vi "Text control 2 v1.8.vi"() -> ()   [LabVIEW 2016]
panel:
  in  "byte count":u32=64
  in  "Serial Settings:Serial End Mode for Reads":u16(ring)=2 items=["None", "LastBit", "TermChar"]
  in  "Timeout (ms)":u32=10000
  in  "Enable Termination\nChar (T)":bool=TRUE
  in  "Termination char\n(0xA = '\\n' = LF)\n(0xD = '\\r' = CR)":u8=13 format="%.0x"
  in  "flow control":u16(ring) items=["None"=0, "XON/XOFF"=1, "RTS/CTS"=2, "DTR/DSR"=4]
  in  "stop bits":u16(ring)=10 items=["1.0"=10, "1.5"=15, "2.0"=20]
  in  "parity":u16(ring) items=["None", "Odd", "Even", "Mark", "Space"]
  in  "data bits":u16=8 min=5 max=8 step=1
  in  "VISA resource name":refnum<visa-resource-name>="COM6"
  in  "baud rate":u32=9600
  out "Serial output":string
  out "error out":errorcluster
  in  "Units":bool
  out "Elapsed Time":dbl caption="Elapsed Time (s)"
  out "Ion vs time":cluster{"Y data in":dbl[], "X data in":dbl[]}[](graph)
  out "Ig":dbl format="%.2e"
  out "Id":dbl format="%.2e"
  out "Is":dbl format="%.2e"
  out "I vs Vg":cluster{"Y data in":dbl[], "X data in":dbl[]}[](graph)
  in  "Panel Controls 2":T1={"Emergency Stop"=refnum, "TransGraph Max"=1e-05, "Text/Graph (text=false)"=TRUE, "TransGraph Min"=1e-11} {"TransGraph Min" format="%.2e"; "TransGraph Max" format="%.2e"}
  out "Currently running:":string="#output s 0 0 0 -0.008 0.008 0.002"
  out "Lines left to run:":string
  in  "Standby":T2
  in  "Full Reset":bool
  in  "SMU4":cluster{"on/off":bool, "Voltage":dbl} {"Voltage" min=-100.0 max=100.0 format="%.2f"}
  in  "Source/Drain Range":u8(slide)=6 max=11 scale=0.0..11.0
  in  "Source/Drain\nRange mode":u16(ring) items=["Auto", "Limited", "Fixed"]
  in  "Gate Range":u8(slide)=6 max=11 scale=0.0..11.0
  in  "Gate Range\nmode":u16(ring) items=["Auto", "Limited", "Fixed"]
  in  "Gate":T3={"Gate Start"=0.0, "Gate Stop"=2.0, "Gate Step (linear only)"=1.0, "Gate Compliance"=0.0001, "Gate PComp"=0.0, "Range mode"=0, "Range"=6} {"Range" max=11 scale=0.0..11.0; "Range mode" items=["Auto", "Limited", "Fixed"]; "Gate PComp" format="%^.2e"; "Gate Compliance" format="%^.2e"; "Gate Step (linear only)" format="%^.4e"; "Gate Stop" format="%^.4e"; "Gate Start" format="%^.4e"}
  in  "Drain 2":T4={"Drain Start"=0.0, "Drain Stop"=2.0, "Drain Compliance"=0.0001, "Drain Step"=1.0, "Drain PComp"=0.0, "Range mode"=0, "Range"=6} {"Range" max=11 scale=0.0..11.0; "Range mode" items=["Auto", "Limited", "Fixed"]; "Drain PComp" format="%^.2e"; "Drain Step" format="%^.4e"; "Drain Compliance" format="%^.2e"; "Drain Stop" format="%^.4e"; "Drain Start" format="%^.4e"}
  in  "Timings 2":T5={"integration time"=0, "Short/Long integration time"=0.00064, "hold time (sec)"=0.0, "delay time (sec)"=0.0, "Step Time (0 disables)"=0.0, "sweep method"=0, "Pulse period"=0.005, "Base voltage"=0.0, "Pulse width"=0.0005} {"Pulse width" min=0.0005 max=0.1 step=0.0001 format="%.4f"; "Base voltage" format="%^.4e"; "Pulse period" min=0.005 max=1.0 step=0.0001 format="%.4f"; "sweep method" items=["Continuous", "Pulsed"]; "Step Time (0 disables)" format="%.2f"; "delay time (sec)" format="%.4f"; "hold time (sec)" format="%.4f"; "Short/Long integration time" format="%^.0e"; "integration time" scale=0.0..2.0}
  in  "Panel Controls":T6={"Emergency Stop"=refnum, "TransGraph Max"=1e-05, "Text/Graph (text=false)"=TRUE} {"TransGraph Max" format="%.2e"}
  in  "Interrupt run":bool
  in  "Drain: Compliance":dbl=0.001 format="%.8f"
  in  "Gate: Compliance":dbl=0.001 format="%.8f"
  out "Path":path=path "C:/users/rlp38/09Apr2009LTtesting/test2.txt"
  in  "hold time /s":dbl format="%.2f"
  in  "delay time /s":dbl format="%.2f"
  in  "integration time":u32(slide) max=2 step=1 scale=0.0..2.0
  in  "Integration time (short)":dbl=0.0019 min=8e-05 max=0.0019 step=8e-05 format="%^.0e"
  in  "Integration time (long)":dbl=0.32 min=0.04 max=2.0 step=0.02 format="%.2f"
  in  "Step delay /s":dbl format="%.2f"
  in  "Program":string="#pulsedstressV d 0.03 20 0 0.5 0.0827 5\n#\n#itime s\n#gaterangemode l\n#drainrangemode l\n#pulsed on 0.05 0 0.02\n#transfer d 1 -1 -0.1 -1 -1 0\n#wait-min 1\n#transfer d 1 -1 -0.1 -1 -1 0\n#output d 0 -1 -0.5 0 -1 -0.1\n#transfer d -10 40 1 5 40 35\n#transfer d -10 40 1 5 40 35\n#output d 0 40 20 0 40 1\n#\n#\n#sample 1 0.008 221 6 0.003\n#samplei 400e-6 200 6 0.002 0.1\n#vsu2pulse -10 4\n#\n#stressV 0.016 0.03 2e-4 0.1e-3 11\n#stressI 220e-7 0.08 15\n#transfer s -1 1 0.5 -0.005 0.005 0.005\n#output s 0 0 0 -0.008 0.008 0.002\n"
  # "Syntax:\nitime [s|m|l]\ngaterangemode [a|l|f]\ndrainrangemode [a|l|f]\npulsed [on|off] PulsePeriod(sec) PulseBaseVoltage PulseONWidth(sec)\nstandby [on l off]\nwait NumMilliseconds\nwait-min NumMinutes\n# texthere = comment\ntransfer [s|d] VgStart VgStop VgStep VdStart VdStop VdStep\noutput [s|d] VgStart VgStop VgStep VdStart VdStop VdStep\nsample Vg Vd NumSamples Time(s) SampleInterval(s)\nsamplei Idg NumSamples Time(s) SampleInterval(s) VDGcompliance\n# if in doubt use SampleInterval(s) = 0.004\nstressV VG VD IGcompliance IDcompliance Duration(sec)\nstressI IDG VDGcompliance Duration(sec)\nvsu2pulse Bias Duration(s)\npulsedstressV [s|d] VEstop VgON VgOFF Period(s) PulseONwidth(s) Vd\nsample-fpp Vg Vd NumSamples Time\nresample-fpp Vg Vd\ntransfer-fpp [s|d] VgStart VgStop VgStep VdStart VdStop VdStep\noutput-fpp [s|d] VgStart VgStop VgStep VdStart VdStop VdStep\nserial SerialPortCommand"
  # "Time"
  # "Sec"
  # "Min"
  # "100 samples is approx 13s with medium integration"
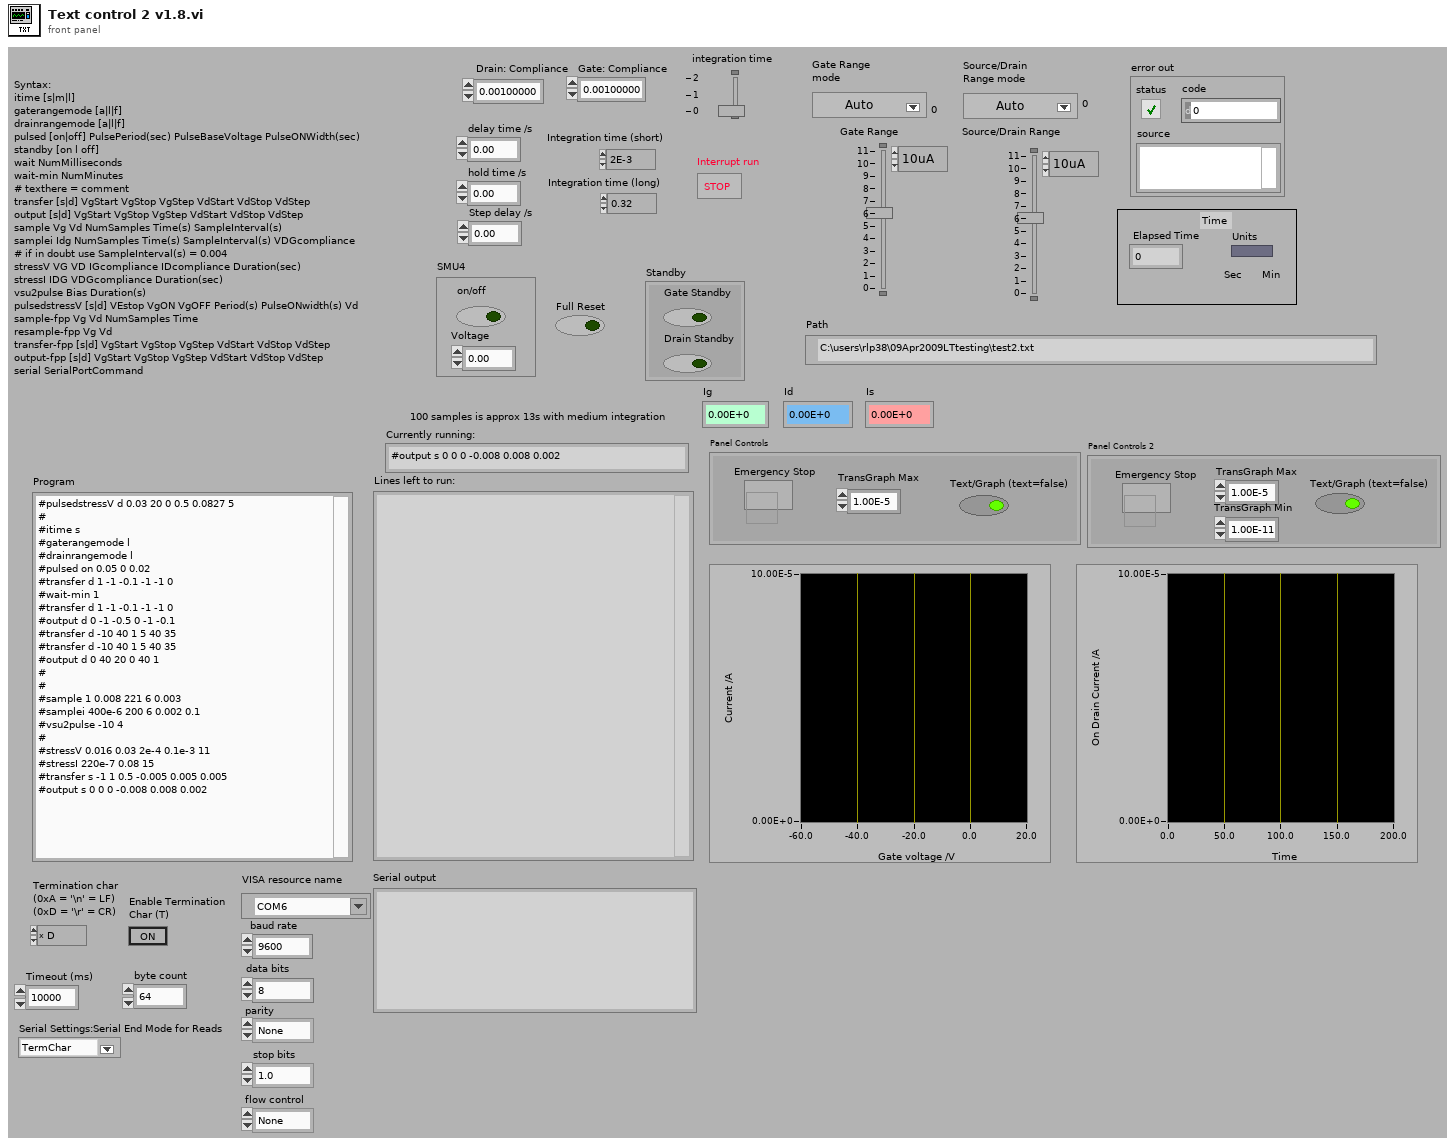
[diagram p1: front panel]
types:
  T1 = cluster{"Emergency Stop":refnum<vi>, "TransGraph Max":dbl, "Text/Graph (text=false)":bool, "TransGraph Min":dbl}
  T2 = cluster{"Gate Standby":bool, "Drain Standby":bool}
  T3 = cluster{"Gate Start":dbl, "Gate Stop":dbl, "Gate Step (linear only)":dbl, "Gate Compliance":dbl, "Gate PComp":dbl, "Range mode":u16, "Range":u8}
  T4 = cluster{"Drain Start":dbl, "Drain Stop":dbl, "Drain Compliance":dbl, "Drain Step":dbl, "Drain PComp":dbl, "Range mode":u16, "Range":u8}
  T5 = cluster{"integration time":u32, "Short/Long integration time":dbl, "hold time (sec)":dbl, "delay time (sec)":dbl, "Step Time (0 disables)":dbl, "sweep method":u16, "Pulse period":dbl, "Base voltage":dbl, "Pulse width":dbl}
  T6 = cluster{"Emergency Stop":refnum<vi>, "TransGraph Max":dbl, "Text/Graph (text=false)":bool}
  T7 = enum16{"open", "replace", "create", "open or create", "replace or create", "replace or create with confirmation"}
  T8 = cluster{"V2 Start":dbl, "V2 Step":dbl, "Number of points":i32}
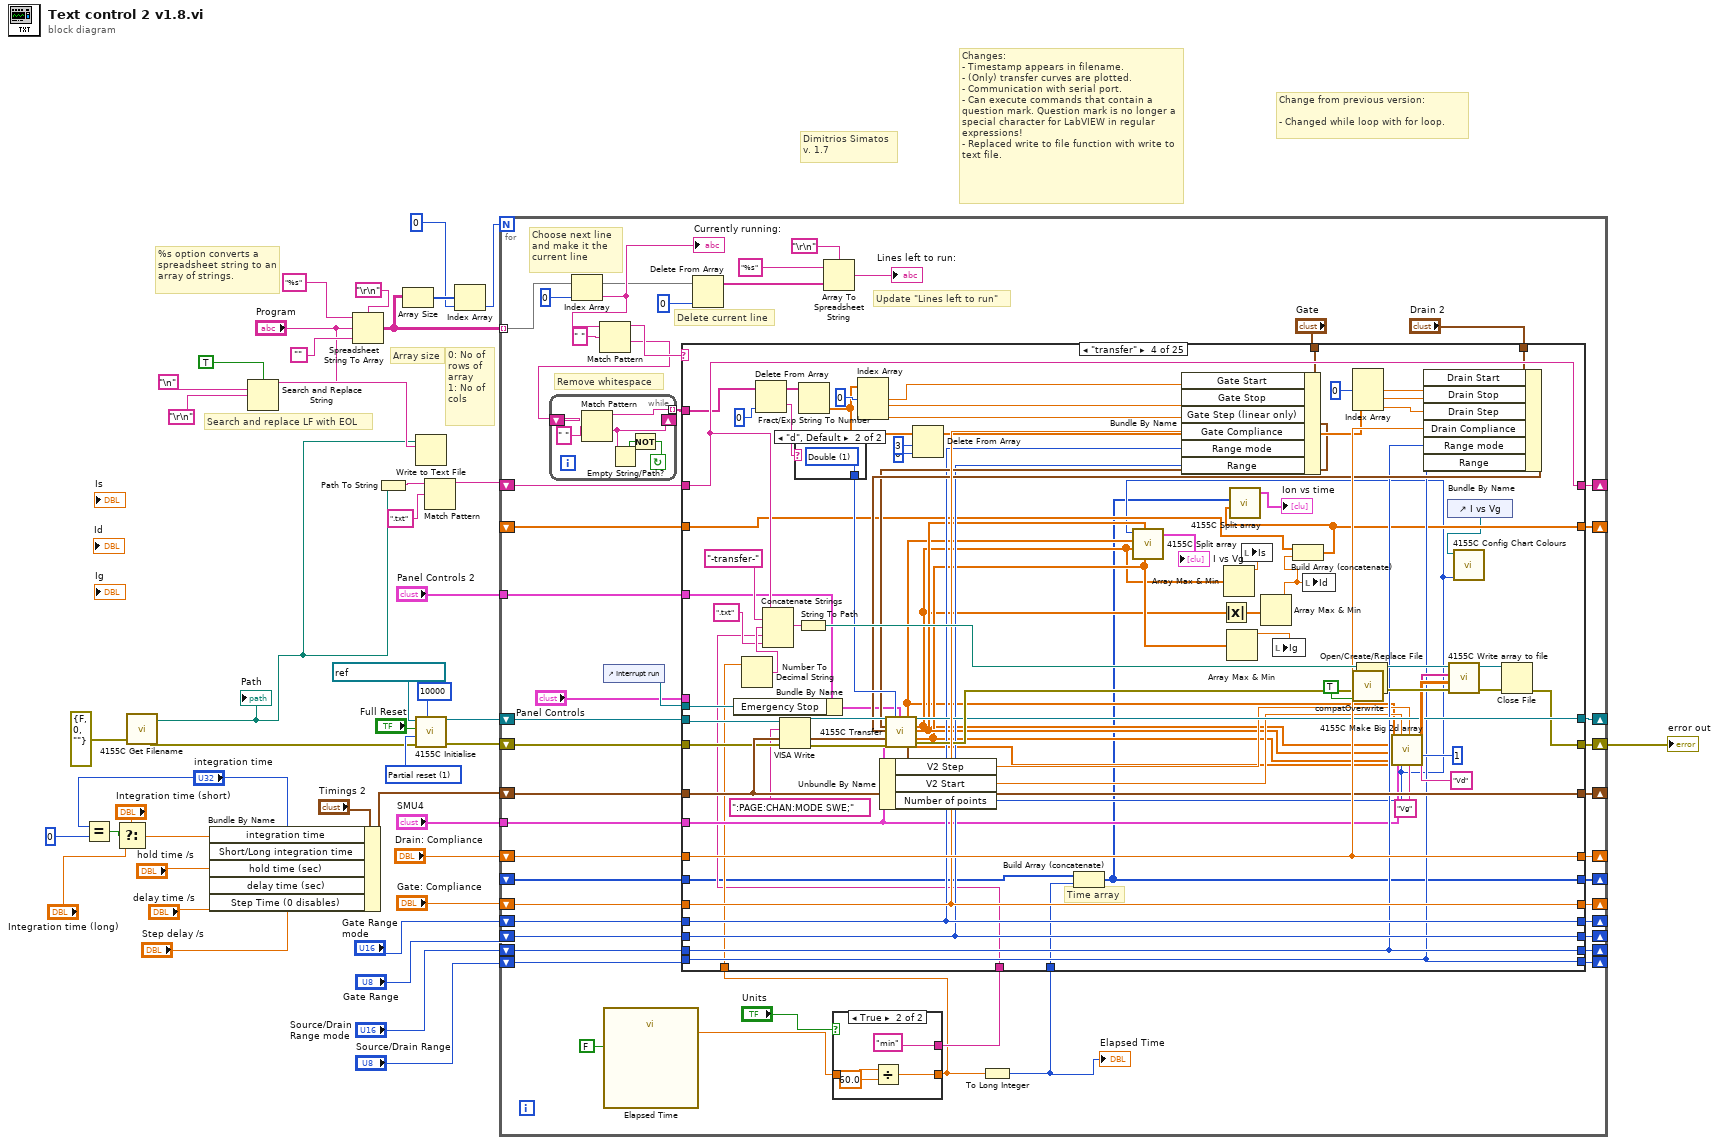
[diagram p0: block diagram]
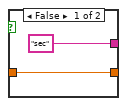
[diagram p2: hidden frame]
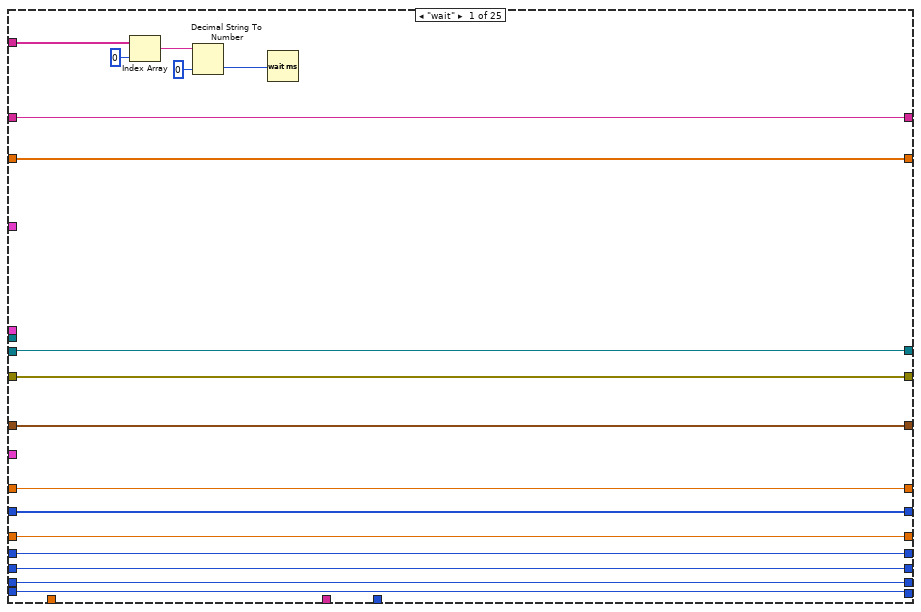
[diagram p3: hidden frame]
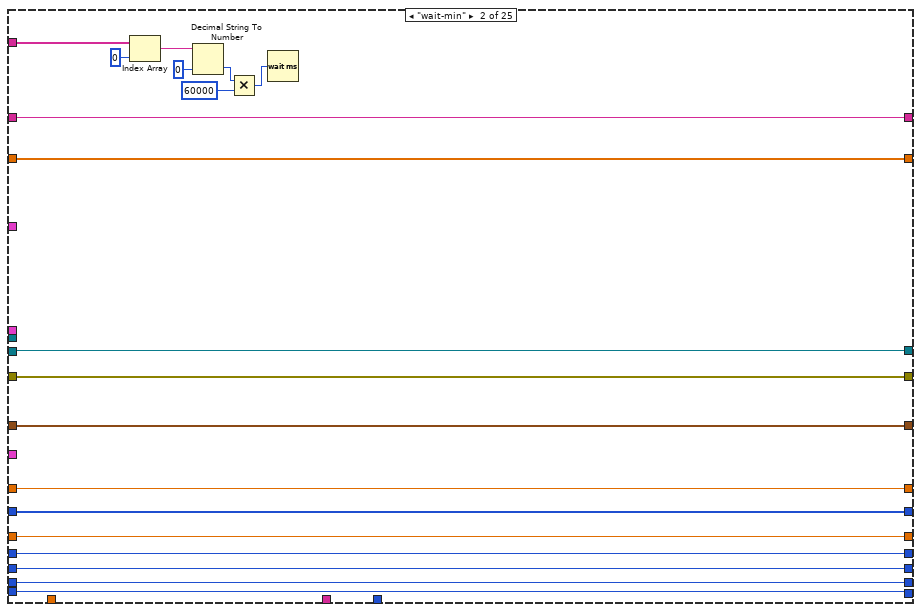
[diagram p4: hidden frame]
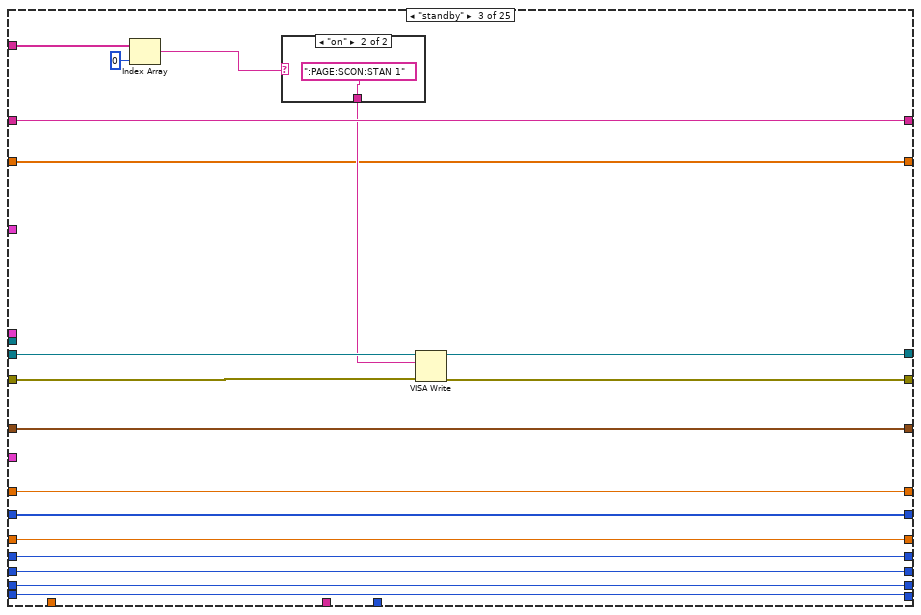
[diagram p5: hidden frame]
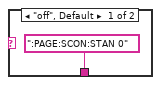
[diagram p6: hidden frame]
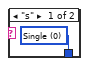
[diagram p7: hidden frame]
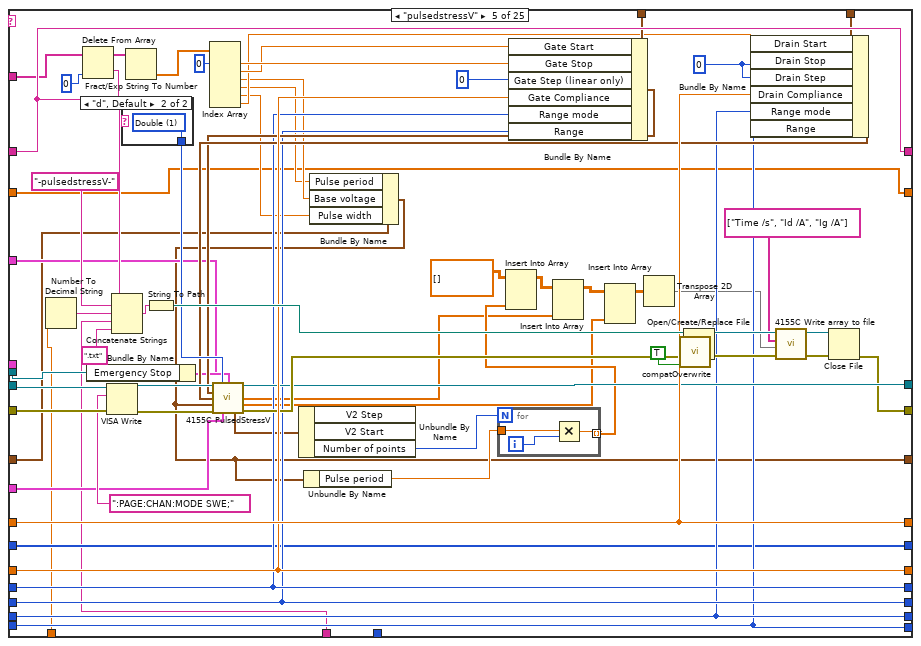
[diagram p8: hidden frame]
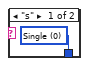
[diagram p9: hidden frame]
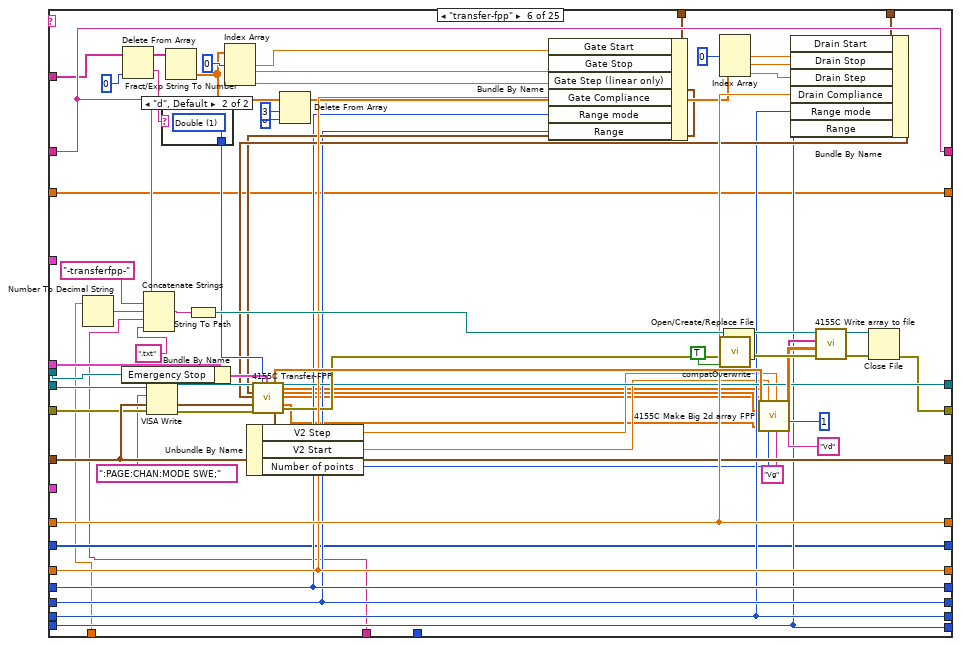
[diagram p10: hidden frame]
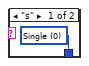
[diagram p11: hidden frame]
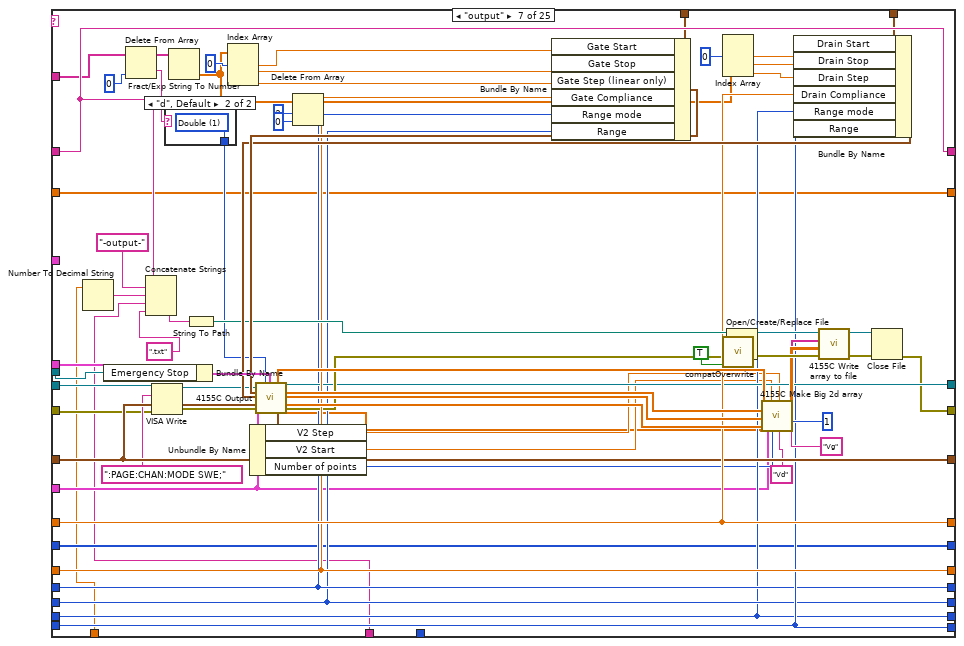
[diagram p12: hidden frame]
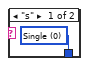
[diagram p13: hidden frame]
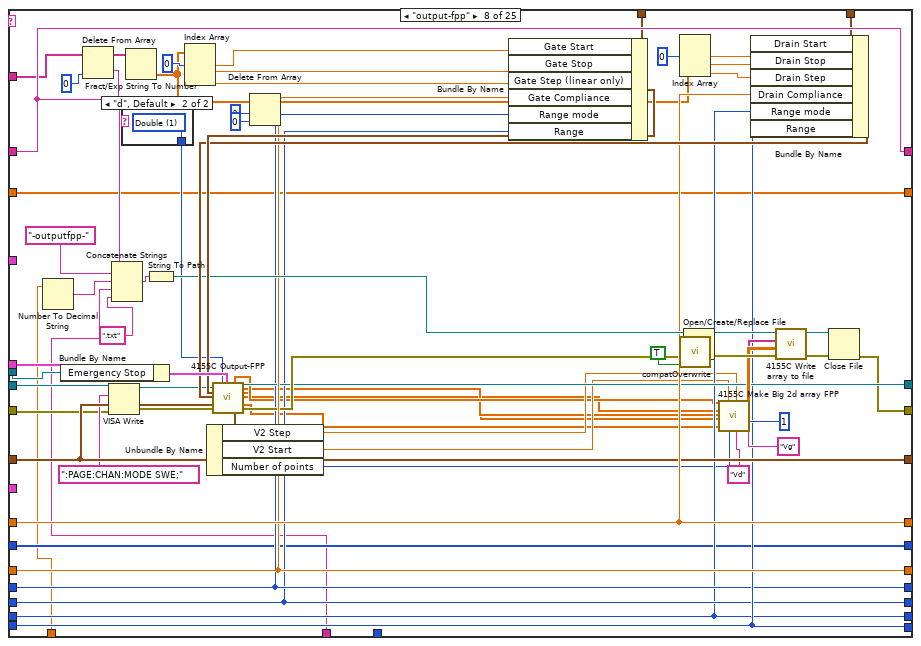
[diagram p14: hidden frame]
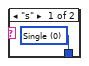
[diagram p15: hidden frame]
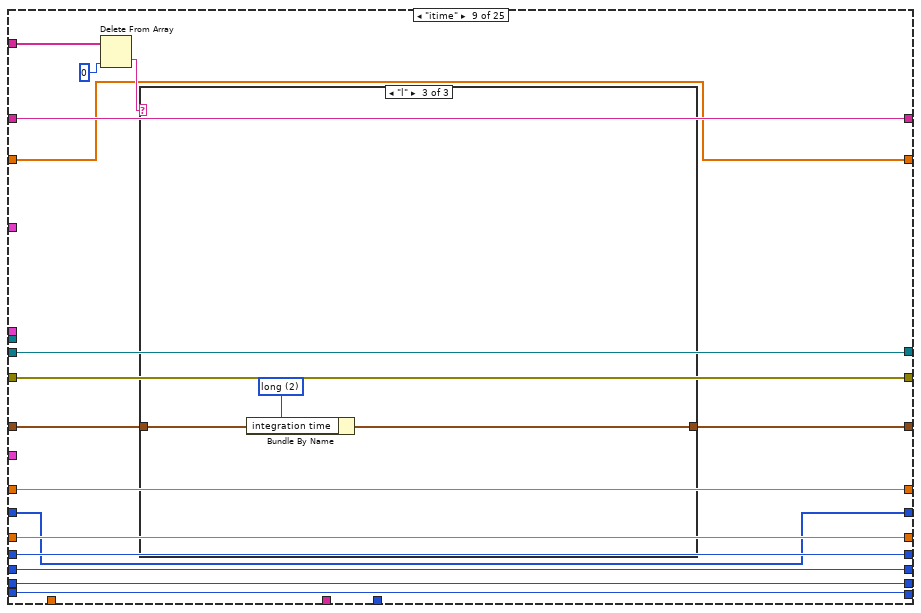
[diagram p16: hidden frame]
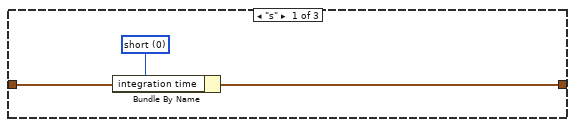
[diagram p17: hidden frame]
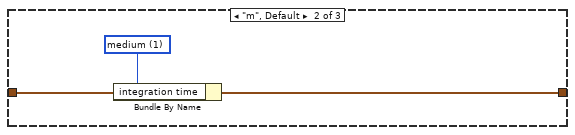
[diagram p18: hidden frame]
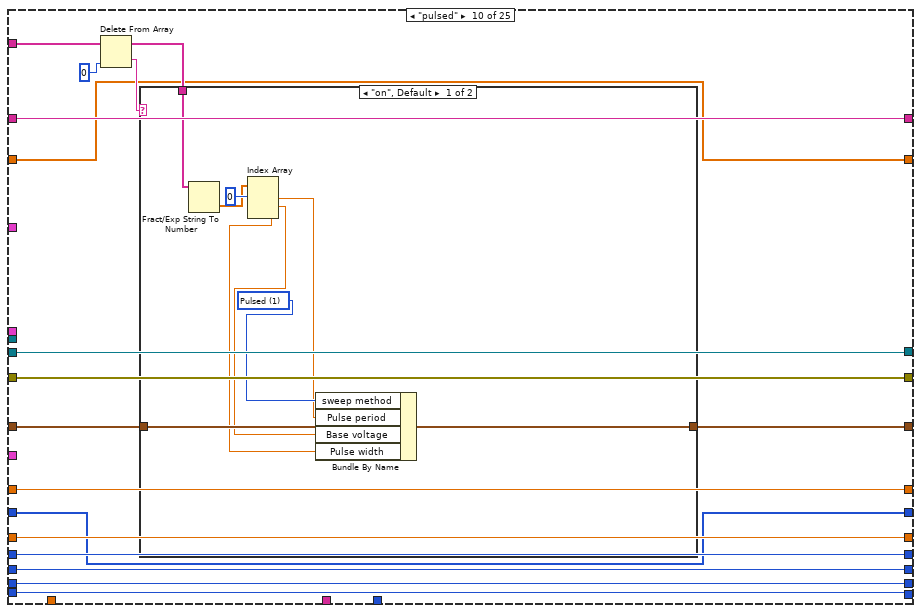
[diagram p19: hidden frame]
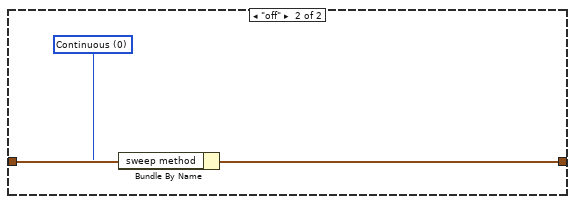
[diagram p20: hidden frame]
diagram:
  w35 = u16 1 items=["Reset All", "Partial reset"] ("Type of reset")
  # "Array size"
  # "%s option converts a spreadsheet string to an array of strings."
  # "0: No of rows of array\n1: No of cols"
  # "Change from previous version:\n\n- Changed while loop with for loop."
  # "Dimitrios Simatos\nv. 1.7"
  # "Changes:\n- Timestamp appears in filename.\n- (Only) transfer curves are plotted.\n- Communication with serial port.\n- Can execute commands that contain a question mark. Question mark is no longer a special character for LabVIEW in regular expressions!\n- Replaced write to file function with write to text file."
  # "Search and replace LF with EOL"
  n1 = Equal?(x="integration time", y=u32 0) -> (x = y?=w39:bool)
  n2 = Select(t="Integration time (short)", s=w39, f="Integration time (long)") -> (s? t:f=w43:dbl)
  n3 = call "4155C Get Filename.vi"("error in (no error)"=errorcluster {"status"=FALSE, "code"=0, "source"=""}) -> ("error out"=w30:errorcluster, "path"=w14:path)  [unwired: 2 in, 1 out]
  "Path" <- w14
  n4 = Bundle By Name(cluster="Timings 2", "integration time"="integration time", "Short/Long integration time"=w43, "hold time (sec)"="hold time /s", "delay time (sec)"="delay time /s", "Step Time (0 disables)"="Step delay /s") -> (w27:T5)
  n5 = Search and Replace String(replace all?=TRUE ("replace all? (F)"), input string="Program", search string="\n", replace string="\r\n") -> (result string=w17:string)  [unwired: 4 in, 3 out]
  n6 = Spreadsheet String To Array(delimiter (Tab)="\r\n", format string="%s", spreadsheet string="Program", array type (2D Dbl)="") -> (array=w2:string[][])
  n7 = Path To String(path=w14) -> (string=w13:string)
  n8 = Array Size(array=w2) -> (size(s)=w7:i32[])
  n9 = Write to Text File(file (use dialog)=w14, text=w17) -> ()  [unwired: 2 in, 3 out]
  n10 = call "4155C Initialise.vi"("VISA resource name in"=refnum<visa-resource-name> "GPIB0::14::INSTR", "Reset"="Full Reset", "Type of reset"=w35, "error in (no error)"=w30, "VISA Timeout Value"=u32 10000) -> ("VISA Resource Name out"=w29:refnum<visa-resource-name>, "error out"=w28:errorcluster)
  n11 = Match Pattern(string=w13, regular expression=".txt") -> (before substring=w12:string)  [unwired: 1 in, 3 out]
  n12 = Index Array(array=w7, index=0) -> (element=w5:i32)
  n13 = for {
    N: w5 -> [_]
    tunnel: "SMU4" -> [w64]
    shift-left: "Source/Drain Range" -> [w69]
    shift-right: [w65] -> _
    shift-left: "Source/Drain\nRange mode" -> [w70]
    shift-right: [w66] -> _
    shift-left: "Gate Range" -> [w71]
    shift-right: [w67] -> _
    shift-left: "Gate Range\nmode" -> [w72]
    shift-right: [w68] -> _
    shift-left: "Gate: Compliance" -> [w83]
    shift-right: [w78] -> _
    shift-left: "Drain: Compliance" -> [w84]
    shift-right: [w79] -> _
    shift-left: w27 -> [w85]
    shift-right: [w80] -> _
    shift-left: w28 -> [w86]
    shift-right: [w81] -> w9
    shift-left: w29 -> [w87]
    shift-right: [w82] -> _
    shift-left: w12 -> [w88]
    shift-right: [w77] -> _
    tunnel: "Panel Controls 2" -> [w63]
    shift-right: [w62] -> _
    shift-left: _ -> [w61]
    shift-right: [w56] -> _
    shift-left: _ -> [w55]
    tunnel: w2 -> [w51] mode=indexing
    # "Choose next line\nand make it the current line"
    # "Delete current line"
    # "Remove whitespace"
    # "Update \"Lines left to run\""
    n14 = Index Array(array=w51, index=0 ("line index")) -> (element=w52:string)
    "Currently running:" <- w52
    n15 = Match Pattern(string=w52, regular expression=" ") -> (before substring=w91:string, after substring=w90:string)  [unwired: 1 in, 2 out]
    n16 = while {
      tunnel: [w99] -> w89 mode=indexing
      shift-left: w90 -> [w101]
      shift-right: [w100] -> _
      stop <- w103 continue-if-true
      n17 = Match Pattern(string=w101, regular expression=" ") -> (before substring=w99:string, after substring=w100:string)  [unwired: 1 in, 2 out]
      n18 = Empty String/Path?(string/path=w100) -> (empty?=w104:bool)
      n19 = Not(x=w104) -> (.not. x?=w103:bool)
    }
    n20 = control-ref of="Interrupt run"() -> (w76:refnum<vi>)
    n21 = call "Elapsed Time"("Auto Reset"=FALSE) -> ("Elapsed Time (s)"=w57:dbl)  [unwired: 11 in, 7 out]
    n22 = Delete From Array(array=w51, index=0) -> (array with subset deleted=w50:string[])  [unwired: 1 in, 1 out]
    n23 = Array To Spreadsheet String(delimiter (Tab)="\r\n", array=w50, 3:"%s" ("format string")) -> (spreadsheet string=→"Lines left to run:":string)
    n24 = case shown="True" "Units" {
      tunnel: ["sec" "min"] -> w58
      tunnel: [w93 w97] -> w54
      tunnel: w57 -> [w93 w96]
      frame False {
      }
      frame True {
        n25 = Divide(x=w96, y=60.0) -> (x/y=w97:dbl)
      }
    }
    n26 = To Long Integer(number=w54) -> (32bit integer=w53:i32)
    "Elapsed Time" <- w53
    n27 = case shown="\"transfer\"" w91 {
      tunnel: w89 -> [w121 w140 w158 w222 w293 w362 w429 w504 w542 w568 w595 w620 w641 w655 _ _ w759 w820 _ w885 w929 w971 w1041 w1103 w1110]
      tunnel: w88 -> [w116 w136 w156 w230 w300 w370 w437 w512 w531 w557 w587 w613 w635 w648 w667 w709 w737 w802 w833 w872 w916 w959 w1035 w1099 w1112]
      tunnel: w87 -> [w115 w135 w147 w200 w284 w339 w405 w480 w532 w558 w588 w614 w636 w649 w672 w711 w765 w826 w837 w891 w935 w977 w1047 w1057 w1116]
      tunnel: w86 -> [w114 w134 w146 w199 w283 w338 w402 w477 w533 w559 w589 w615 w637 w650 w671 w682 w764 w825 w836 w890 w934 w976 w1046 w1056 w1115]
      tunnel: w85 -> [w113 w133 w155 w226 w259 w366 w433 w508 w541 w567 w586 w612 w634 w647 w670 w706 w728 w794 w842 w865 w909 w952 w1034 w1098 w1117]
      tunnel: w84 -> [w112 w132 w154 w228 w298 w368 w435 w510 w540 w566 w594 w619 w640 w654 w669 w691 w763 w824 w845 w889 w933 w975 w1045 w1107 w1118]
      tunnel: w83 -> [w111 w131 w153 w227 w297 w367 w434 w509 w539 w565 w593 w618 w639 w653 w668 w692 w738 w803 w844 w873 w917 w960 w1036 w1100 w1120]
      tunnel: [w115 w135 w145 w224 w295 w364 w431 w506 w532 w558 w588 w614 w636 w649 w672 w711 w729 w776 w835 w866 w910 w953 w987 w1059 w1116] -> w82
      tunnel: [w114 w134 w144 w223 w294 w363 w430 w505 w533 w559 w589 w615 w637 w650 w671 w681 w739 w777 w834 w874 w918 w961 w986 w1058 w1114] -> w81
      tunnel: [w113 w133 w155 w226 w255 w366 w433 w508 w534 w560 w586 w612 w634 w647 w670 w706 w728 w794 w842 w865 w909 w952 w1034 w1098 w1117] -> w80
      tunnel: [w112 w132 w154 w228 w298 w368 w435 w510 w540 w566 w594 w619 w640 w654 w669 w691 w763 w824 w845 w889 w933 w975 w1045 w1107 w1118] -> w79
      tunnel: [w111 w131 w153 w227 w297 w367 w434 w509 w539 w565 w593 w618 w639 w653 w668 w692 w738 w803 w844 w873 w917 w960 w1036 w1100 w1120] -> w78
      tunnel: [w116 w136 w156 w230 w300 w370 w437 w512 w531 w557 w587 w613 w635 w648 w667 w709 w737 w802 w833 w872 w916 w959 w1035 w1099 w1112] -> w77
      tunnel: w76 -> [_ _ _ w233 w304 w375 w445 w516 _ _ _ _ _ _ _ _ w734 w799 _ w871 w915 w958 w1007 w1075 _]
      tunnel: "Gate" -> [_ _ _ w209 w287 w349 w416 w491 _ _ _ _ _ _ _ _ _ _ _ _ _ _ _ _ _]
      tunnel: "Drain 2" -> [_ _ _ w208 w286 w348 w415 w490 _ _ _ _ _ _ _ _ _ _ _ _ _ _ _ _ _]
      tunnel: "Panel Controls" -> [_ _ _ _ _ w347 w414 w489 _ _ _ _ _ _ _ _ _ _ _ _ _ _ _ _ _]
      tunnel: w72 -> [w110 w130 w152 w193 w277 w332 w400 w475 w538 w564 _ w611 w633 w646 w666 w693 w724 w790 w838 w861 w905 w948 w1030 w1094 w1121]
      tunnel: w71 -> [w109 w129 w151 w192 w276 w331 w399 w474 w537 w563 w592 _ w624 w652 w665 w694 w725 w791 w839 w862 w906 w949 w1031 w1095 w1122]
      tunnel: w70 -> [w108 w128 w150 w191 w275 w330 w398 w473 w536 w562 w591 w617 w638 _ w664 w695 w726 w792 w840 w863 w907 w950 w1032 w1096 w1123]
      tunnel: w69 -> [w107 w127 w149 w190 w274 w329 w401 w476 w535 w561 w590 w616 _ w651 w663 w696 w727 w793 w841 w864 w908 w951 w1033 w1097 w1124]
      tunnel: [w110 w130 w152 w193 w277 w332 w400 w475 w538 w564 w585 w611 w633 w646 w666 w693 w724 w790 w838 w861 w905 w948 w1030 w1094 w1121] -> w68
      tunnel: [w109 w129 w151 w192 w276 w331 w399 w474 w537 w563 w592 w603 w624 w652 w665 w694 w725 w791 w839 w862 w906 w949 w1031 w1095 w1122] -> w67
      tunnel: [w108 w128 w150 w191 w275 w330 w398 w473 w536 w562 w591 w617 w638 w645 w664 w695 w726 w792 w840 w863 w907 w950 w1032 w1096 w1123] -> w66
      tunnel: [w107 w127 w149 w190 w274 w329 w401 w476 w535 w561 w590 w616 w625 w651 w663 w696 w727 w793 w841 w864 w908 w951 w1033 w1097 w1124] -> w65
      tunnel: w64 -> [_ _ _ w185 w271 _ w393 _ _ _ _ _ _ _ _ _ _ _ _ _ _ _ _ _ _]
      tunnel: w63 -> [_ _ _ w183 w270 _ _ _ _ _ _ _ _ _ _ _ _ _ _ _ _ _ _ _ _]
      tunnel: [w106 w123 w142 w172 w247 w319 w390 w462 w530 w555 w584 w602 w623 w644 w662 w677 w716 w774 w832 w850 w898 w942 w984 w1052 w1113] -> w62
      tunnel: w61 -> [w106 w123 w142 w171 w247 w319 w390 w462 w530 w555 w584 w602 w623 w644 w662 w677 w716 w774 w832 w850 w898 w942 w984 w1052 w1113]
      tunnel: w54 -> [_ _ _ w167 w244 w317 w387 w459 _ _ _ _ _ _ _ w675 w714 w771 _ w847 w895 w939 w981 w1048 _]
      tunnel: w58 -> [_ _ _ w164 w243 w315 w386 w458 _ _ _ _ _ _ _ w673 w712 w770 _ w846 w894 w938 w980 w1049 _]
      tunnel: w53 -> [_ _ _ w161 _ _ _ _ _ _ _ _ _ _ _ _ _ _ _ _ _ _ _ _ _]
      tunnel: [w105 w122 w141 w163 w246 w318 w389 w461 w529 w554 w583 w601 w622 w643 w661 w676 w715 w773 w831 w849 w897 w941 w983 w1051 w1119] -> w56
      tunnel: w55 -> [w105 w122 w141 w162 w246 w318 w389 w461 w529 w554 w583 w601 w622 w643 w661 w676 w715 w773 w831 w849 w897 w941 w983 w1051 w1119]
      frame "wait" {
        n28 = Index Array(array=w121, index=0 ("Index")) -> (element=w119:string)
        n29 = Decimal String To Number(string=w119, default (0L)=u32 0) -> (number=w118:u32)  [unwired: 1 in, 1 out]
        n30 = Wait (ms)(milliseconds to wait=w118) -> ()  [unwired: 1 out]
      }
      frame "wait-min" {
        n31 = Index Array(array=w140, index=0 ("Index")) -> (element=w138:string)
        n32 = Decimal String To Number(string=w138, default (0L)=u32 0) -> (number=w126:u32)  [unwired: 1 in, 1 out]
        n33 = Multiply(x=w126, y=u32 60000) -> (x*y=w125:u32)
        n34 = Wait (ms)(milliseconds to wait=w125) -> ()  [unwired: 1 out]
      }
      frame "standby" {
        n35 = Index Array(array=w158, index=0 ("Index")) -> (element=w148:string)
        n36 = case shown="\"on\"" w148 {
          tunnel: [":PAGE:SCON:STAN 0" ":PAGE:SCON:STAN 1"] -> w143
          frame "off", Default {
          }
          frame "on" {
          }
        }
        n37 = VISA Write(VISA resource name=w147, write buffer=w143, error in (no error)=w146) -> (VISA resource name out=w145:refnum<visa-resource-name>, error out=w144:errorcluster)  [unwired: 1 out]
      }
      frame "transfer" {
        # "Time array"
        n38 = Bundle By Name(cluster=w183, "Emergency Stop"=w233) -> (w184:T1)
        n39 = Number To Decimal String(number=w167) -> (decimal integer string=w166:string)  [unwired: 1 in]
        n40 = Delete From Array(array=w222, index=0 ("Index")) -> (deleted portion=w220:string, array with subset deleted=w219:string[])  [unwired: 1 in]
        n41 = Concatenate Strings(w230, "-transfer-" ("Prefix"), w166, w164, ".txt" ("Suffix")) -> (w232:string)
        n42 = VISA Write(VISA resource name=w200, write buffer=":PAGE:CHAN:MODE SWE;" ("write buffer (\"\")"), error in (no error)=w199) -> (VISA resource name out=w197:refnum<visa-resource-name>, error out=w198:errorcluster)  [unwired: 1 out]
        n43 = case shown="\"d\", Default" w220 {
          tunnel: [w241 w242] -> w218
          frame "s" {
            w241 = u16 0 items=["Single", "Double"] ("sweep mode")
          }
          frame "d", Default {
            w242 = u16 1 items=["Single", "Double"] ("sweep mode")
          }
        }
        n44 = String To Path(string=w232) -> (path=w229:path)
        n45 = Fract/Exp String To Number(string=w219) -> (number=w204:dbl[])  [unwired: 3 in, 1 out]
        n46 = Index Array(array=w204, index #1=0 ("Index")) -> (element #1=w217:dbl, element #2=w216:dbl, element #3=w215:dbl)  [unwired: 2 in]
        n47 = Delete From Array(array=w204, length=3 ("Length"), index=0 ("Index")) -> (array with subset deleted=w202:dbl[])  [unwired: 1 out]
        n48 = Build Array (concatenate)(w162, w161) -> (w163:i32[])
        n49 = Bundle By Name(cluster=w209, "Gate Start"=w217, "Gate Stop"=w216, "Gate Step (linear only)"=w215, "Gate Compliance"=w227, "Range mode"=w193, "Range"=w192) -> (w194:T3)
        n50 = Index Array(array=w202, index #1=0 ("Index")) -> (element #1=w212:dbl, element #2=w211:dbl, element #3=w210:dbl)  [unwired: 2 in]
        n51 = call <vilib>:"compatOverwrite.vi"("overwrite (F)"=TRUE) -> ("overwrite?"=w182:T7)
        n52 = Bundle By Name(cluster=w208, "Drain Start"=w212, "Drain Stop"=w211, "Drain Step"=w210, "Drain Compliance"=w228, "Range mode"=w191, "Range"=w190) -> (w195:T4)
        n53 = call "4155C Transfer.vi"("VISA resource name in"=w197, "Gate"=w194, "Drain"=w195, "Timings"=w226, "error in (no error)"=w198, "SMU4"=w185, "sweep mode"=w218, "Panel Controls"=w184) -> ("VG"=w173:dbl[], "Outparams"=w189:T8, "VISA Resource Name out"=w224:refnum<visa-resource-name>, "IS"=w175:dbl[], "ID"=w180:dbl[], "IG"=w176:dbl[], "error out"=w225:errorcluster, "SMU4"=w186:dbl[])  [unwired: 12 in]
        n54 = Unbundle By Name(w189) -> ("V2 Step"=w188:dbl, "V2 Start"=w187:dbl, "Number of points"=w169:i32)
        n55 = call "4155C Split array.vi"("Number of VAR2 steps"=w169, "Y2 data in"=w180, "X data in"=w173, "Y1 data in"=w175, "Y3 data in"=w176) -> ("Array of clusters"=→"I vs Vg":cluster{"Y data in":dbl[], "X data in":dbl[]}[])  [unwired: 2 in, 1 out]
        n56 = Absolute Value(x=w175) -> (abs(x)=w179:dbl[])
        n57 = Array Max & Min(array=w175) -> (max value=w177:dbl)  [unwired: 3 out]
        n58 = Array Max & Min(array=w176) -> (max value=w178:dbl)  [unwired: 3 out]
        n59 = local write "Is"(w177) -> ()
        n60 = Array Max & Min(array=w179) -> (max value=w170:dbl)  [unwired: 3 out]
        n61 = local write "Ig"(w178) -> ()
        n62 = Build Array (concatenate)(w171, w170) -> (w172:dbl[])
        n63 = call "4155C Split array.vi"("X data in"=w163, "Y1 data in"=w172) -> ("Array of clusters"=→"Ion vs time":cluster{"Y data in":dbl[], "X data in":dbl[]}[])  [unwired: 5 in, 1 out]
        n64 = local write "Id"(w170) -> ()
        n65 = Open/Create/Replace File(file path (use dialog)=w229, error in=w225, operation (0:open)=w182) -> (refnum out=w238:refnum<file>, error out=w239:errorcluster)  [unwired: 3 in, 1 out]
        n66 = call "4155C Make Big 2d array.vi"("1D Var1"=w173, "1d IS"=w175, "1d ID"=w180, "1d IG"=w176, "1d SMU4"=w186, "SMU4"=w185, "VAR2 START"=w187, "Number of VAR2 steps"=w169, "VAR2 STEP"=w188, "VAR1 Name"="Vg", "Decimal places in header"=i8 1, "VAR2 Name"="Vd") -> ("Header array"=w234:string[], "Data array"=w235:dbl[][])  [unwired: 14 in]
        n67 = control-ref of="I vs Vg"() -> (w168:refnum<vi>)
        n68 = call "4155C Write array to file.vi"("Byte Stream File Refnum"=w238, "Header"=w234, "Data Array"=w235, "error in (no error)"=w239) -> ("dup refnum"=w236:refnum<file>, "error out"=w237:errorcluster)  [unwired: 1 in]
        n69 = call "4155C Config Chart Colours.vi"("Numeric"=w169, "XY Graph 2"=w168) -> ()  [unwired: 6 in]
        n70 = Close File(refnum=w236, error in=w237) -> (error out=w223:errorcluster)  [unwired: 1 out]
      }
      frame "pulsedstressV" {
        w253 = 0
        n71 = Number To Decimal String(number=w244) -> (decimal integer string=w301:string)  [unwired: 1 in]
        n72 = Delete From Array(array=w293, index=0 ("Index")) -> (deleted portion=w291:string, array with subset deleted=w290:string[])  [unwired: 1 in]
        n73 = Bundle By Name(cluster=w270, "Emergency Stop"=w304) -> (w272:T1)
        n74 = VISA Write(VISA resource name=w284, write buffer=":PAGE:CHAN:MODE SWE;" ("write buffer (\"\")"), error in (no error)=w283) -> (VISA resource name out=w281:refnum<visa-resource-name>, error out=w282:errorcluster)  [unwired: 1 out]
        n75 = Concatenate Strings(w300, "-pulsedstressV-" ("Substring"), w301, w243, ".txt" ("Substring")) -> (w303:string)
        n76 = case shown="\"d\", Default" w291 {
          tunnel: [w313 w314] -> w289
          frame "s" {
            w313 = u16 0 items=["Single", "Double"] ("sweep mode")
          }
          frame "d", Default {
            w314 = u16 1 items=["Single", "Double"] ("sweep mode")
          }
        }
        n77 = Fract/Exp String To Number(string=w290) -> (number=w285:dbl[])  [unwired: 3 in, 1 out]
        n78 = String To Path(string=w303) -> (path=w299:path)
        n79 = Index Array(array=w285, index #1=0 ("Index")) -> (element #1=w262:dbl, element #2=w261:dbl, element #3=w258:dbl, element #4=w257:dbl, element #5=w256:dbl, element #6=w260:dbl)  [unwired: 5 in]
        n80 = Bundle By Name(cluster=w259, "Pulse period"=w257, "Base voltage"=w258, "Pulse width"=w256) -> (w255:T5)
        n81 = Unbundle By Name(w255) -> ("Pulse period"=w263:dbl)
        n82 = Bundle By Name(cluster=w287, "Gate Start"=w261, "Gate Stop"=w262, "Gate Step (linear only)"=0, "Gate Compliance"=w297, "Range mode"=w277, "Range"=w276) -> (w278:T3)
        n83 = call <vilib>:"compatOverwrite.vi"("overwrite (F)"=TRUE) -> ("overwrite?"=w248:T7)
        n84 = Bundle By Name(cluster=w286, "Drain Start"=w260, "Drain Stop"=w253, "Drain Step"=w253, "Drain Compliance"=w298, "Range mode"=w275, "Range"=w274) -> (w279:T4)
        n85 = call "4155C PulsedStressV.vi"("VISA resource name in"=w281, "sweep mode"=w289, "Panel Controls"=w272, "Gate"=w278, "Drain"=w279, "Timings"=w255, "error in (no error)"=w282, "SMU4"=w271) -> ("VISA Resource Name out"=w295:refnum<visa-resource-name>, "ID"=w251:dbl[], "IG"=w249:dbl[], "Outparams"=w273:T8, "error out"=w296:errorcluster)  [unwired: 3 in]
        n86 = Unbundle By Name(w273) -> ("Number of points"=w250:i32)  [unwired: 2 out]
        n87 = for {
          N: w250 -> [_]
          tunnel: [w310] -> w252 mode=indexing
          tunnel: w263 -> [w312]
          i -> [w311]
          n88 = Multiply(x=w312, y=w311) -> (x*y=w310:dbl)
        }
        n89 = Insert Into Array(array=dbl[][] [] ("Input Array"), new element=w252) -> (w264:dbl[][])  [unwired: 2 in]
        n90 = Insert Into Array(array=w264, new element=w251) -> (w269:dbl[][])  [unwired: 2 in]
        n91 = Insert Into Array(array=w269, new element=w249) -> (w268:dbl[][])  [unwired: 2 in]
        n92 = Transpose 2D Array(2D array=w268) -> (transposed array=w267:dbl[][])
        n93 = Open/Create/Replace File(file path (use dialog)=w299, error in=w296, operation (0:open)=w248) -> (refnum out=w307:refnum<file>, error out=w308:errorcluster)  [unwired: 3 in, 1 out]
        n94 = call "4155C Write array to file.vi"("Byte Stream File Refnum"=w307, "Header"=string[] ["Time /s", "Id /A", "Ig /A"], "Data Array"=w267, "error in (no error)"=w308) -> ("dup refnum"=w305:refnum<file>, "error out"=w306:errorcluster)  [unwired: 1 in]
        n95 = Close File(refnum=w305, error in=w306) -> (error out=w294:errorcluster)  [unwired: 1 out]
      }
      frame "transfer-fpp" {
        n96 = Number To Decimal String(number=w317) -> (decimal integer string=w371:string)  [unwired: 1 in]
        n97 = Bundle By Name(cluster=w347, "Emergency Stop"=w375) -> (w383:T6)
        n98 = Delete From Array(array=w362, index=0 ("Index")) -> (deleted portion=w360:string, array with subset deleted=w359:string[])  [unwired: 1 in]
        n99 = Concatenate Strings(w370, "-transferfpp-" ("Substring"), w371, w315, ".txt" ("Substring")) -> (w373:string)
        n100 = VISA Write(VISA resource name=w339, write buffer=":PAGE:CHAN:MODE SWE;" ("write buffer (\"\")"), error in (no error)=w338) -> (VISA resource name out=w336:refnum<visa-resource-name>, error out=w337:errorcluster)  [unwired: 1 out]
        n101 = case shown="\"d\", Default" w360 {
          tunnel: [w384 w385] -> w358
          frame "s" {
            w384 = u16 0 items=["Single", "Double"] ("sweep mode")
          }
          frame "d", Default {
            w385 = u16 1 items=["Single", "Double"] ("sweep mode")
          }
        }
        n102 = Fract/Exp String To Number(string=w359) -> (number=w343:dbl[])  [unwired: 3 in, 1 out]
        n103 = String To Path(string=w373) -> (path=w369:path)
        n104 = Index Array(array=w343, index #1=0 ("Index")) -> (element #1=w357:dbl, element #2=w356:dbl, element #3=w355:dbl)  [unwired: 2 in]
        n105 = Delete From Array(array=w343, length=3 ("Length"), index=0 ("Index")) -> (array with subset deleted=w341:dbl[])  [unwired: 1 out]
        n106 = Bundle By Name(cluster=w349, "Gate Start"=w357, "Gate Stop"=w356, "Gate Step (linear only)"=w355, "Gate Compliance"=w367, "Range mode"=w332, "Range"=w331) -> (w333:T3)
        n107 = Index Array(array=w341, index #1=0 ("Index")) -> (element #1=w352:dbl, element #2=w351:dbl, element #3=w350:dbl)  [unwired: 2 in]
        n108 = call <vilib>:"compatOverwrite.vi"("overwrite (F)"=TRUE) -> ("overwrite?"=w320:T7)
        n109 = Bundle By Name(cluster=w348, "Drain Start"=w352, "Drain Stop"=w351, "Drain Step"=w350, "Drain Compliance"=w368, "Range mode"=w330, "Range"=w329) -> (w334:T4)
        n110 = call "4155C Transfer-FPP.vi"("VISA resource name in"=w336, "Gate"=w333, "Drain"=w334, "Timings"=w366, "error in (no error)"=w337, "sweep mode"=w358, "Panel Controls"=w383) -> ("VG"=w374:dbl[], "Outparams"=w328:T8, "VISA Resource Name out"=w364:refnum<visa-resource-name>, "Vprobe2"=w324:dbl[], "ID"=w323:dbl[], "IG"=w322:dbl[], "Vprobe1"=w321:dbl[], "error out"=w365:errorcluster)  [unwired: 13 in]
        n111 = Unbundle By Name(w328) -> ("V2 Step"=w327:dbl, "V2 Start"=w326:dbl, "Number of points"=w325:i32)
        n112 = Open/Create/Replace File(file path (use dialog)=w369, error in=w365, operation (0:open)=w320) -> (refnum out=w380:refnum<file>, error out=w381:errorcluster)  [unwired: 3 in, 1 out]
        n113 = call "4155C Make Big 2d array FPP.vi"("1D Var1"=w374, "1d ID"=w323, "1d Vp2"=w324, "1d IG"=w322, "1d Vp1"=w321, "VAR2 START"=w326, "Number of VAR2 steps"=w325, "VAR2 STEP"=w327, "VAR1 Name"="Vg", "Decimal places in header"=i8 1, "VAR2 Name"="Vd") -> ("Header array"=w376:string[], "Data array"=w377:dbl[][])  [unwired: 15 in]
        n114 = call "4155C Write array to file.vi"("Byte Stream File Refnum"=w380, "Header"=w376, "Data Array"=w377, "error in (no error)"=w381) -> ("dup refnum"=w378:refnum<file>, "error out"=w379:errorcluster)  [unwired: 1 in]
        n115 = Close File(refnum=w378, error in=w379) -> (error out=w363:errorcluster)  [unwired: 1 out]
      }
      frame "output" {
        n116 = Number To Decimal String(number=w387) -> (decimal integer string=w438:string)  [unwired: 1 in]
        n117 = Bundle By Name(cluster=w414, "Emergency Stop"=w445) -> (w455:T6)
        n118 = Delete From Array(array=w429, index=0 ("Index")) -> (deleted portion=w427:string, array with subset deleted=w426:string[])  [unwired: 1 in]
        n119 = Concatenate Strings(w437, "-output-" ("Substring"), w438, w386, ".txt" ("Substring")) -> (w440:string)
        n120 = VISA Write(VISA resource name=w405, write buffer=":PAGE:CHAN:MODE SWE;" ("write buffer (\"\")"), error in (no error)=w402) -> (VISA resource name out=w404:refnum<visa-resource-name>, error out=w403:errorcluster)  [unwired: 1 out]
        n121 = case shown="\"d\", Default" w427 {
          tunnel: [w456 w457] -> w425
          frame "s" {
            w456 = u16 0 items=["Single", "Double"] ("sweep mode")
          }
          frame "d", Default {
            w457 = u16 1 items=["Single", "Double"] ("sweep mode")
          }
        }
        n122 = Fract/Exp String To Number(string=w426) -> (number=w408:dbl[])  [unwired: 3 in, 1 out]
        n123 = String To Path(string=w440) -> (path=w436:path)
        n124 = Index Array(array=w408, index #1=0 ("Index")) -> (element #1=w424:dbl, element #2=w423:dbl, element #3=w422:dbl)  [unwired: 2 in]
        n125 = Delete From Array(array=w408, length=3 ("Length"), index=0 ("Index")) -> (array with subset deleted=w407:dbl[])  [unwired: 1 out]
        n126 = Bundle By Name(cluster=w416, "Gate Start"=w424, "Gate Stop"=w423, "Gate Step (linear only)"=w422, "Gate Compliance"=w434, "Range mode"=w400, "Range"=w399) -> (w454:T3)
        n127 = Index Array(array=w407, index #1=0 ("Index")) -> (element #1=w419:dbl, element #2=w418:dbl, element #3=w417:dbl)  [unwired: 2 in]
        n128 = call <vilib>:"compatOverwrite.vi"("overwrite (F)"=TRUE) -> ("overwrite?"=w391:T7)
        n129 = Bundle By Name(cluster=w415, "Drain Start"=w419, "Drain Stop"=w418, "Drain Step"=w417, "Drain Compliance"=w435, "Range mode"=w398, "Range"=w401) -> (w453:T4)
        n130 = call "4155C Output.vi"("VISA resource name in"=w404, "Gate"=w454, "Drain"=w453, "Timings"=w433, "error in (no error)"=w403, "SMU4"=w393, "sweep mode"=w425, "Panel controls"=w455) -> ("VD"=w441:dbl[], "Outparams"=w396:T8, "VISA Resource Name out"=w431:refnum<visa-resource-name>, "IS"=w444:dbl[], "ID"=w443:dbl[], "IG"=w442:dbl[], "error out"=w432:errorcluster, "SMU4"=w392:dbl[])  [unwired: 12 in]
        n131 = Unbundle By Name(w396) -> ("V2 Step"=w397:dbl, "V2 Start"=w395:dbl, "Number of points"=w394:i32)
        n132 = Open/Create/Replace File(file path (use dialog)=w436, error in=w432, operation (0:open)=w391) -> (refnum out=w450:refnum<file>, error out=w451:errorcluster)  [unwired: 3 in, 1 out]
        n133 = call "4155C Make Big 2d array.vi"("1D Var1"=w441, "1d IS"=w444, "1d ID"=w443, "1d IG"=w442, "1d SMU4"=w392, "SMU4"=w393, "VAR2 START"=w395, "Number of VAR2 steps"=w394, "VAR2 STEP"=w397, "VAR1 Name"="Vd", "Decimal places in header"=i8 1, "VAR2 Name"="Vg") -> ("Header array"=w446:string[], "Data array"=w447:dbl[][])  [unwired: 14 in]
        n134 = call "4155C Write array to file.vi"("Byte Stream File Refnum"=w450, "Header"=w446, "Data Array"=w447, "error in (no error)"=w451) -> ("dup refnum"=w448:refnum<file>, "error out"=w449:errorcluster)  [unwired: 1 in]
        n135 = Close File(refnum=w448, error in=w449) -> (error out=w430:errorcluster)  [unwired: 1 out]
      }
      frame "output-fpp" {
        n136 = Number To Decimal String(number=w459) -> (decimal integer string=w513:string)  [unwired: 1 in]
        n137 = Bundle By Name(cluster=w489, "Emergency Stop"=w516) -> (w526:T6)
        n138 = Delete From Array(array=w504, index=0 ("Index")) -> (deleted portion=w502:string, array with subset deleted=w501:string[])  [unwired: 1 in]
        n139 = VISA Write(VISA resource name=w480, write buffer=":PAGE:CHAN:MODE SWE;" ("write buffer (\"\")"), error in (no error)=w477) -> (VISA resource name out=w479:refnum<visa-resource-name>, error out=w478:errorcluster)  [unwired: 1 out]
        n140 = Concatenate Strings(w512, "-outputfpp-" ("Substring"), w513, w458, ".txt" ("Substring")) -> (w515:string)
        n141 = case shown="\"d\", Default" w502 {
          tunnel: [w527 w528] -> w500
          frame "s" {
            w527 = u16 0 items=["Single", "Double"] ("sweep mode")
          }
          frame "d", Default {
            w528 = u16 1 items=["Single", "Double"] ("sweep mode")
          }
        }
        n142 = Fract/Exp String To Number(string=w501) -> (number=w483:dbl[])  [unwired: 3 in, 1 out]
        n143 = String To Path(string=w515) -> (path=w511:path)
        n144 = Index Array(array=w483, index #1=0 ("Index")) -> (element #1=w499:dbl, element #2=w498:dbl, element #3=w497:dbl)  [unwired: 2 in]
        n145 = Delete From Array(array=w483, length=3 ("Length"), index=0 ("Index")) -> (array with subset deleted=w482:dbl[])  [unwired: 1 out]
        n146 = Bundle By Name(cluster=w491, "Gate Start"=w499, "Gate Stop"=w498, "Gate Step (linear only)"=w497, "Gate Compliance"=w509, "Range mode"=w475, "Range"=w474) -> (w525:T3)
        n147 = Index Array(array=w482, index #1=0 ("Index")) -> (element #1=w494:dbl, element #2=w493:dbl, element #3=w492:dbl)  [unwired: 2 in]
        n148 = call <vilib>:"compatOverwrite.vi"("overwrite (F)"=TRUE) -> ("overwrite?"=w463:T7)
        n149 = Bundle By Name(cluster=w490, "Drain Start"=w494, "Drain Stop"=w493, "Drain Step"=w492, "Drain Compliance"=w510, "Range mode"=w473, "Range"=w476) -> (w524:T4)
        n150 = call "4155C Output-FPP.vi"("VISA resource name in"=w479, "Gate"=w525, "Drain"=w524, "Timings"=w508, "error in (no error)"=w478, "sweep mode"=w500, "Panel controls"=w526) -> ("VD"=w468:dbl[], "Outparams"=w471:T8, "VISA Resource Name out"=w506:refnum<visa-resource-name>, "Vprobe2"=w467:dbl[], "ID"=w466:dbl[], "IG"=w465:dbl[], "Vprobe1"=w464:dbl[], "error out"=w507:errorcluster)  [unwired: 13 in]
        n151 = Unbundle By Name(w471) -> ("V2 Step"=w472:dbl, "V2 Start"=w470:dbl, "Number of points"=w469:i32)
        n152 = Open/Create/Replace File(file path (use dialog)=w511, error in=w507, operation (0:open)=w463) -> (refnum out=w521:refnum<file>, error out=w522:errorcluster)  [unwired: 3 in, 1 out]
        n153 = call "4155C Make Big 2d array FPP.vi"("1D Var1"=w468, "1d ID"=w466, "1d Vp2"=w467, "1d IG"=w465, "1d Vp1"=w464, "VAR2 START"=w470, "Number of VAR2 steps"=w469, "VAR2 STEP"=w472, "VAR1 Name"="Vd", "Decimal places in header"=i8 1, "VAR2 Name"="Vg") -> ("Header array"=w517:string[], "Data array"=w518:dbl[][])  [unwired: 15 in]
        n154 = call "4155C Write array to file.vi"("Byte Stream File Refnum"=w521, "Header"=w517, "Data Array"=w518, "error in (no error)"=w522) -> ("dup refnum"=w519:refnum<file>, "error out"=w520:errorcluster)  [unwired: 1 in]
        n155 = Close File(refnum=w519, error in=w520) -> (error out=w505:errorcluster)  [unwired: 1 out]
      }
      frame "itime" {
        n156 = Delete From Array(array=w542, index=0 ("Index")) -> (deleted portion=w543:string)  [unwired: 1 in, 1 out]
        n157 = case shown="\"l\"" w543 {
          tunnel: w541 -> [w547 w549 w552]
          tunnel: [w546 w548 w551] -> w534
          frame "s" {
            w545 = u32 0 items=["short  ", "medium  ", "long  "] ("integration time 2")
            n158 = Bundle By Name(cluster=w547, "integration time"=w545) -> (w546:T5)
          }
          frame "m", Default {
            w550 = u32 1 items=["short  ", "medium  ", "long  "] ("integration time 2")
            n159 = Bundle By Name(cluster=w549, "integration time"=w550) -> (w548:T5)
          }
          frame "l" {
            w553 = u32 2 items=["short  ", "medium  ", "long  "] ("integration time 2")
            n160 = Bundle By Name(cluster=w552, "integration time"=w553) -> (w551:T5)
          }
        }
      }
      frame "pulsed" {
        n161 = Delete From Array(array=w568, index=0 ("Index")) -> (deleted portion=w569:string, array with subset deleted=w556:string[])  [unwired: 1 in]
        n162 = case shown="\"on\", Default" w569 {
          tunnel: w567 -> [w579 w582]
          tunnel: [w578 w581] -> w560
          tunnel: w556 -> [w576 _]
          frame "on", Default {
            w577 = u16 1 items=["Continuous", "Pulsed"] ("sweep method")
            n163 = Fract/Exp String To Number(string=w576) -> (number=w574:dbl[])  [unwired: 3 in, 1 out]
            n164 = Index Array(array=w574, index #1=0 ("Index")) -> (element #1=w573:dbl, element #2=w572:dbl, element #3=w571:dbl)  [unwired: 2 in]
            n165 = Bundle By Name(cluster=w579, "sweep method"=w577, "Pulse period"=w573, "Base voltage"=w572, "Pulse width"=w571) -> (w578:T5)
          }
          frame "off" {
            w580 = u16 0 items=["Continuous", "Pulsed"] ("sweep method")
            n166 = Bundle By Name(cluster=w582, "sweep method"=w580) -> (w581:T5)
          }
        }
      }
      frame "gaterangemode" {
        n167 = Delete From Array(array=w595, index=0 ("Index")) -> (deleted portion=w596:string)  [unwired: 1 in, 1 out]
        n168 = case shown="\"f\"" w596 {
          tunnel: [w598 w599 w600] -> w585
          frame "a", Default {
            w598 = u16 0 items=["Auto", "Limited", "Fixed"] ("Gate Range\nmode 2")
          }
          frame "f" {
            w599 = u16 2 items=["Auto", "Limited", "Fixed"] ("Gate Range\nmode 2")
          }
          frame "l" {
            w600 = u16 1 items=["Auto", "Limited", "Fixed"] ("Gate Range\nmode 2")
          }
        }
      }
      frame "gaterange" {
        (unwired) u8 11 items=["10fA  ", "100fA  ", "1nA  ", "10nA", "100nA", "1uA", "10uA", "100uA", "1mA", "10mA", "100mA", "1A"] ("Gate Range 2")
        n169 = Delete From Array(array=w620, index=0 ("Index")) -> (deleted portion=w610:string)  [unwired: 1 in, 1 out]
        n170 = Scan Value(string=w610, format string="") -> (value=w608:dbl)  [unwired: 1 in, 1 out]
        n171 = Logarithm Base 10(1:w608) -> (0:w607:dbl)
        n172 = Round To Nearest(number=w607) -> (nearest integer value=w606:dbl)
        n173 = Add(x=w606, y=11.0) -> (x+y=w604:dbl)
        n174 = To Unsigned Byte Integer(number=w604) -> (unsigned 8bit integer=w603:u8)
      }
      frame "drainrange" {
        (unwired) u8 11 items=["10fA  ", "100fA  ", "1nA  ", "10nA", "100nA", "1uA", "10uA", "100uA", "1mA", "10mA", "100mA", "1A"] ("Gate Range 2")
        n175 = Delete From Array(array=w641, index=0 ("Index")) -> (deleted portion=w632:string)  [unwired: 1 in, 1 out]
        n176 = Scan Value(string=w632, format string="") -> (value=w630:dbl)  [unwired: 1 in, 1 out]
        n177 = Logarithm Base 10(1:w630) -> (0:w629:dbl)
        n178 = Round To Nearest(number=w629) -> (nearest integer value=w628:dbl)
        n179 = Add(x=w628, y=11.0) -> (x+y=w626:dbl)
        n180 = To Unsigned Byte Integer(number=w626) -> (unsigned 8bit integer=w625:u8)
      }
      frame "drainrangemode" {
        n181 = Delete From Array(array=w655, index=0 ("Index")) -> (deleted portion=w656:string)  [unwired: 1 in, 1 out]
        n182 = case shown="\"f\"" w656 {
          tunnel: [w658 w659 w660] -> w645
          frame "a", Default {
            w658 = u16 0 items=["Auto", "Limited", "Fixed"] ("Gate Range\nmode 2")
          }
          frame "f" {
            w659 = u16 2 items=["Auto", "Limited", "Fixed"] ("Gate Range\nmode 2")
          }
          frame "l" {
            w660 = u16 1 items=["Auto", "Limited", "Fixed"] ("Gate Range\nmode 2")
          }
        }
      }
      frame "Error", Default {
      }
      frame "logfile" {
        n183 = Number To Decimal String(number=w675) -> (decimal integer string=w710:string)  [unwired: 1 in]
        n184 = Concatenate Strings(w709, "logfile" ("Substring"), w710, w673, ".txt" ("Substring")) -> (w707:string)
        n185 = String To Path(string=w707) -> (path=w680:path)
        n186 = Unbundle(w706) -> ("integration time"=w705:u32, "Short/Long integration time"=w704:dbl, "hold time (sec)"=w703:dbl, "delay time (sec)"=w702:dbl, "Step Time (0 disables)"=w701:dbl, "sweep method"=w700:u16, "Pulse period"=w699:dbl, "Base voltage"=w698:dbl, "Pulse width"=w697:dbl)
        n187 = Build Array(w705, w704, w703, w702, w701, w700, w699, w698, w697, w691, w692, w693, w694, w695, w696) -> (w684:dbl[])
        n188 = Insert Into Array(array=dbl[][] [] ("Input Array"), new element=w684) -> (w683:dbl[][])  [unwired: 2 in]
        n189 = call <vilib>:"compatOverwrite.vi"("overwrite (F)"=TRUE) -> ("overwrite?"=w678:T7)
        n190 = Open/Create/Replace File(file path (use dialog)=w680, error in=w682, operation (0:open)=w678) -> (refnum out=w688:refnum<file>, error out=w687:errorcluster)  [unwired: 3 in, 1 out]
        n191 = call "4155C Write array to file.vi"("Byte Stream File Refnum"=w688, "Header"=string[] ["Int Time", "Short/Long Itime", "Hold time", "Delay time", "Step time", "Sweep method", "Pulse period", "Base Voltage", "Pulse width", "Drain compliance", "Gate compliance", "Gate range mode", "Gate range", "S/D range mode", "S/D range"], "Data Array"=w683, "error in (no error)"=w687) -> ("dup refnum"=w690:refnum<file>, "error out"=w689:errorcluster)  [unwired: 1 in]
        n192 = Close File(refnum=w690, error in=w689) -> (error out=w681:errorcluster)  [unwired: 1 out]
      }
      frame "sample" {
        n193 = Number To Decimal String(number=w714) -> (decimal integer string=w762:string)  [unwired: 1 in]
        n194 = Fract/Exp String To Number(string=w759) -> (number=w720:dbl[])  [unwired: 3 in, 1 out]
        n195 = Concatenate Strings(w737, "-sample-" ("Substring"), w762, w712, ".txt" ("Substring")) -> (w760:string)
        n196 = String To Path(string=w760) -> (path=w741:path)
        n197 = Index Array(array=w720, index=0 ("Index")) -> (element=w757:dbl)
        n198 = Index Array(array=w720, index=2 ("Index")) -> (element=w753:dbl)
        n199 = Index Array(array=w720, index=3 ("Index")) -> (element=w722:dbl)
        n200 = Index Array(array=w720, index=4 ("Index")) -> (element=w719:dbl)
        n201 = call "4155C Config Sampling Measurements.vi"("Sampling interval"=w719, "Sample time"=w722, "Display on/off"=TRUE, "Timings"=w728, "Num Points"=w753, "error in (no error)"=w764, "Drain Compliance"=w763, "Gate Compliance"=w738, "VISA session"=w765) -> ("error out"=w766:errorcluster, "dup VISA resource name"=w767:refnum<visa-resource-name>)  [unwired: 1 in]
        n202 = Index Array(array=w720, index=1 ("Index")) -> (element=w754:dbl)
        n203 = call "4155C Take Sample.vi"("Emergency Stop"=w734, "error in (no error)"=w766, "Vd"=w754, "Vg"=w757, "VISA resource name in"=w767) -> ("error out"=w732:errorcluster, "Id"=w769:dbl[], "Ig"=w743:dbl[], "VISA Resource Name out"=w730:refnum<visa-resource-name>, "Is"=w768:dbl[], "Time"=w747:dbl[])  [unwired: 1 in]
        n204 = Insert Into Array(array=dbl[][] [] ("Input Array"), new element=w747) -> (w746:dbl[][])  [unwired: 2 in]
        n205 = Insert Into Array(array=w746, new element=w743) -> (w745:dbl[][])  [unwired: 2 in]
        n206 = Insert Into Array(array=w745, new element=w769) -> (w744:dbl[][])  [unwired: 2 in]
        n207 = VISA Write(VISA resource name=w730, write buffer=":DISP ON" ("write buffer (\"\")"), error in (no error)=w732) -> (VISA resource name out=w729:refnum<visa-resource-name>, error out=w731:errorcluster)  [unwired: 1 out]
        n208 = Insert Into Array(array=w744, new element=w768) -> (w736:dbl[][])  [unwired: 2 in]
        n209 = Transpose 2D Array(2D array=w736) -> (transposed array=w735:dbl[][])
        n210 = call <vilib>:"compatOverwrite.vi"("overwrite (F)"=TRUE) -> ("overwrite?"=w717:T7)
        n211 = Open/Create/Replace File(file path (use dialog)=w741, error in=w731, operation (0:open)=w717) -> (refnum out=w750:refnum<file>, error out=w749:errorcluster)  [unwired: 3 in, 1 out]
        n212 = call "4155C Write array to file.vi"("Byte Stream File Refnum"=w750, "Header"=string[] ["Time /s", "Ig /A", "Id /A", "Is /A"], "Data Array"=w735, "error in (no error)"=w749) -> ("dup refnum"=w752:refnum<file>, "error out"=w751:errorcluster)  [unwired: 1 in]
        n213 = Close File(refnum=w752, error in=w751) -> (error out=w739:errorcluster)  [unwired: 1 out]
      }
      frame "samplei" {
        n214 = Number To Decimal String(number=w771) -> (decimal integer string=w823:string)  [unwired: 1 in]
        n215 = Fract/Exp String To Number(string=w820) -> (number=w787:dbl[])  [unwired: 3 in, 1 out]
        n216 = Concatenate Strings(w802, "-samplei-" ("Substring"), w823, w770, ".txt" ("Substring")) -> (w821:string)
        n217 = String To Path(string=w821) -> (path=w805:path)
        n218 = Index Array(array=w787, index=4 ("Index")) -> (element=w781:dbl)
        n219 = Index Array(array=w787, index=3 ("Index")) -> (element=w782:dbl)
        n220 = Index Array(array=w787, index=1 ("Index")) -> (element=w784:dbl)
        n221 = Index Array(array=w787, index=0 ("Index")) -> (element=w785:dbl)
        n222 = Index Array(array=w787, index=2 ("Index")) -> (element=w783:dbl)
        n223 = call "4155C Config SamplingI Measurements.vi"("Sample time"=w783, "Display on/off"=TRUE, "Timings"=w794, "Num Points"=w784, "error in (no error)"=w825, "Sampling interval"=w782, "VISA session"=w826) -> ("error out"=w827:errorcluster, "dup VISA resource name"=w828:refnum<visa-resource-name>)  [unwired: 3 in]
        n224 = call "4155C Take SampleI.vi"("Emergency Stop"=w799, "error in (no error)"=w827, "Idg 2"=w785, "Vdg compliance 2"=w781, "VISA resource name in"=w828) -> ("error out"=w797:errorcluster, "Idg"=w830:dbl[], "Vdg"=w807:dbl[], "VISA Resource Name out"=w795:refnum<visa-resource-name>, "Is"=w829:dbl[], "Time"=w811:dbl[])  [unwired: 1 in]
        n225 = Insert Into Array(array=dbl[][] [] ("Input Array"), new element=w811) -> (w810:dbl[][])  [unwired: 2 in]
        n226 = Insert Into Array(array=w810, new element=w807) -> (w809:dbl[][])  [unwired: 2 in]
        n227 = Insert Into Array(array=w809, new element=w830) -> (w808:dbl[][])  [unwired: 2 in]
        n228 = VISA Write(VISA resource name=w795, write buffer=":DISP ON" ("write buffer (\"\")"), error in (no error)=w797) -> (VISA resource name out=w780:refnum<visa-resource-name>, error out=w796:errorcluster)  [unwired: 1 out]
        n229 = Insert Into Array(array=w808, new element=w829) -> (w801:dbl[][])  [unwired: 2 in]
        n230 = Transpose 2D Array(2D array=w801) -> (transposed array=w800:dbl[][])
        n231 = call <vilib>:"compatOverwrite.vi"("overwrite (F)"=TRUE) -> ("overwrite?"=w775:T7)
        n232 = Open/Create/Replace File(file path (use dialog)=w805, error in=w796, operation (0:open)=w775) -> (refnum out=w814:refnum<file>, error out=w813:errorcluster)  [unwired: 3 in, 1 out]
        n233 = call "4155C Write array to file.vi"("Byte Stream File Refnum"=w814, "Header"=string[] ["Time /s", "Vdg /V", "Idg /A", "Is /A"], "Data Array"=w800, "error in (no error)"=w813) -> ("dup refnum"=w816:refnum<file>, "error out"=w815:errorcluster)  [unwired: 1 in]
        n234 = Close File(refnum=w816, error in=w815) -> (error out=w778:errorcluster)  [unwired: 1 out]
        n235 = VISA Write(VISA resource name=w780, write buffer=";:PAGE:SCON:STAN OFF;:PAGE:CHAN:VSU2:DIS;" ("write buffer (\"\")"), error in (no error)=w778) -> (VISA resource name out=w776:refnum<visa-resource-name>, error out=w777:errorcluster)  [unwired: 1 out]
      }
      frame "#" {
        n236 = VISA Write(VISA resource name=w837, write buffer=":DISP ON" ("write buffer (\"\")"), error in (no error)=w836) -> (VISA resource name out=w835:refnum<visa-resource-name>, error out=w834:errorcluster)  [unwired: 1 out]
      }
      frame "stressV" {
        n237 = Number To Decimal String(number=w847) -> (decimal integer string=w888:string)  [unwired: 1 in]
        n238 = Fract/Exp String To Number(string=w885) -> (number=w858:dbl[])  [unwired: 3 in, 1 out]
        n239 = Concatenate Strings(w872, "-stressV-" ("Substring"), w888, w846, ".txt" ("Substring")) -> (w886:string)
        n240 = String To Path(string=w886) -> (path=w876:path)
        n241 = Index Array(array=w858, index=3 ("Index")) -> (element=w855:dbl)
        n242 = Index Array(array=w858, index=1 ("Index")) -> (element=w853:dbl)
        n243 = Index Array(array=w858, index=0 ("Index")) -> (element=w852:dbl)
        n244 = Index Array(array=w858, index=4 ("Index")) -> (element=w857:dbl)
        n245 = Index Array(array=w858, index=2 ("Index")) -> (element=w854:dbl)
        n246 = call "4155C Config V Stress.vi"("VISA session"=w891, "ID compliance"=w855, "VD"=w853, "VG"=w852, "IG compliance"=w854, "error in (no error)"=w890, "Display on/off"=TRUE) -> ("dup VISA resource name"=w893:refnum<visa-resource-name>, "error out"=w892:errorcluster)
        n247 = call "4155C Apply Stress.vi"("error in (no error)"=w892, "Duration"=w857, "Emergency Stop"=w871, "VISA resource name in"=w893) -> ("error out"=w869:errorcluster, "VISA Resource Name out"=w867:refnum<visa-resource-name>)
        n248 = VISA Write(VISA resource name=w867, write buffer=":DISP ON" ("write buffer (\"\")"), error in (no error)=w869) -> (VISA resource name out=w866:refnum<visa-resource-name>, error out=w868:errorcluster)  [unwired: 1 out]
        n249 = call <vilib>:"compatOverwrite.vi"("overwrite (F)"=TRUE) -> ("overwrite?"=w851:T7)
        n250 = Open/Create/Replace File(file path (use dialog)=w876, error in=w868, operation (0:open)=w851) -> (refnum out=w879:refnum<file>, error out=w878:errorcluster)  [unwired: 3 in, 1 out]
        n251 = call "4155C Write array to file.vi"("Byte Stream File Refnum"=w879, "Header"=string[] ["V stress completed successfully", ""], "error in (no error)"=w878) -> ("dup refnum"=w881:refnum<file>, "error out"=w880:errorcluster)  [unwired: 2 in]
        n252 = Close File(refnum=w881, error in=w880) -> (error out=w874:errorcluster)  [unwired: 1 out]
      }
      frame "stressI" {
        n253 = Number To Decimal String(number=w895) -> (decimal integer string=w932:string)  [unwired: 1 in]
        n254 = Fract/Exp String To Number(string=w929) -> (number=w904:dbl[])  [unwired: 3 in, 1 out]
        n255 = Concatenate Strings(w916, "-stressI-" ("Substring"), w932, w894, ".txt" ("Substring")) -> (w930:string)
        n256 = String To Path(string=w930) -> (path=w920:path)
        n257 = Index Array(array=w904, index=1 ("Index")) -> (element=w900:dbl)
        n258 = Index Array(array=w904, index=0 ("Index")) -> (element=w901:dbl)
        n259 = call "4155C Config I Stress.vi"("VISA session"=w935, "IDG"=w901, "VDG compliance"=w900, "error in (no error)"=w934, "Display on/off"=TRUE) -> ("dup VISA resource name"=w937:refnum<visa-resource-name>, "error out"=w936:errorcluster)
        n260 = Index Array(array=w904, index=2 ("Index")) -> (element=w902:dbl)
        n261 = call "4155C Apply Stress.vi"("error in (no error)"=w936, "Duration"=w902, "Emergency Stop"=w915, "VISA resource name in"=w937) -> ("error out"=w913:errorcluster, "VISA Resource Name out"=w911:refnum<visa-resource-name>)
        n262 = VISA Write(VISA resource name=w911, write buffer=":DISP ON" ("write buffer (\"\")"), error in (no error)=w913) -> (VISA resource name out=w910:refnum<visa-resource-name>, error out=w912:errorcluster)  [unwired: 1 out]
        n263 = call <vilib>:"compatOverwrite.vi"("overwrite (F)"=TRUE) -> ("overwrite?"=w899:T7)
        n264 = Open/Create/Replace File(file path (use dialog)=w920, error in=w912, operation (0:open)=w899) -> (refnum out=w923:refnum<file>, error out=w922:errorcluster)  [unwired: 3 in, 1 out]
        n265 = call "4155C Write array to file.vi"("Byte Stream File Refnum"=w923, "Header"=string[] ["I stress completed successfully", ""], "error in (no error)"=w922) -> ("dup refnum"=w925:refnum<file>, "error out"=w924:errorcluster)  [unwired: 2 in]
        n266 = Close File(refnum=w925, error in=w924) -> (error out=w918:errorcluster)  [unwired: 1 out]
      }
      frame "vsu2pulse" {
        n267 = Number To Decimal String(number=w939) -> (decimal integer string=w974:string)  [unwired: 1 in]
        n268 = Fract/Exp String To Number(string=w971) -> (number=w947:dbl[])  [unwired: 3 in, 1 out]
        n269 = Concatenate Strings(w959, "-vsu2-" ("Substring"), w974, w938, ".txt" ("Substring")) -> (w972:string)
        n270 = String To Path(string=w972) -> (path=w963:path)
        n271 = Index Array(array=w947, index=1 ("Index")) -> (element=w946:dbl)
        n272 = Index Array(array=w947, index=0 ("Index")) -> (element=w944:dbl)
        n273 = call "4155C Config VSU2 Stress.vi"("error in (no error)"=w976, "VSU2"=w944, "Display on/off"=TRUE, "VISA session"=w977) -> ("error out"=w978:errorcluster, "dup VISA resource name"=w979:refnum<visa-resource-name>)
        n274 = call "4155C Apply Stress.vi"("error in (no error)"=w978, "Duration"=w946, "Emergency Stop"=w958, "VISA resource name in"=w979) -> ("error out"=w956:errorcluster, "VISA Resource Name out"=w954:refnum<visa-resource-name>)
        n275 = VISA Write(VISA resource name=w954, write buffer=":DISP ON" ("write buffer (\"\")"), error in (no error)=w956) -> (VISA resource name out=w953:refnum<visa-resource-name>, error out=w955:errorcluster)  [unwired: 1 out]
        n276 = call <vilib>:"compatOverwrite.vi"("overwrite (F)"=TRUE) -> ("overwrite?"=w943:T7)
        n277 = Open/Create/Replace File(file path (use dialog)=w963, error in=w955, operation (0:open)=w943) -> (refnum out=w966:refnum<file>, error out=w965:errorcluster)  [unwired: 3 in, 1 out]
        n278 = call "4155C Write array to file.vi"("Byte Stream File Refnum"=w966, "Header"=string[] ["VSU2 pulse completed successfully", ""], "error in (no error)"=w965) -> ("dup refnum"=w968:refnum<file>, "error out"=w967:errorcluster)  [unwired: 2 in]
        n279 = Close File(refnum=w968, error in=w967) -> (error out=w961:errorcluster)  [unwired: 1 out]
      }
      frame "sample-fpp" {
        w992 = string[] ["Time /s", "Id VgVd /A", "Ig VgVd /A", "Vp1 VgVd /V", "Vp2 VgVd /V"] ("Header")
        w996 = "%d" ("format string")
        n280 = Number To Decimal String(number=w981) -> (decimal integer string=w1044:string)  [unwired: 1 in]
        n281 = Fract/Exp String To Number(string=w1041) -> (number=w1029:dbl[])  [unwired: 3 in, 1 out]
        n282 = Concatenate Strings(w1035, "-samplefpp-" ("Substring"), w1044, w980, ".txt" ("Substring")) -> (w1042:string)
        n283 = String To Path(string=w1042) -> (path=w1004:path)
        n284 = Index Array(array=w1029, index=0 ("Index")) -> (element=w990:dbl)
        n285 = Index Array(array=w1029, index=1 ("Index")) -> (element=w989:dbl)
        n286 = Index Array(array=w1029, index=2 ("Index")) -> (element=w1037:dbl)
        n287 = Index Array(array=w1029, index=3 ("Index")) -> (element=w1027:dbl)
        n288 = call "4155C Config Sampling Measurements FPP.vi"("VISA session"=w1047, "Num Points"=w1037, "Vg"=w990, "Display on/off"=TRUE, "Gate Compliance"=w1036, "Drain Compliance"=w1045, "Standby"="Standby", "error in (no error)"=w1046, "Timings"=w1034, "Vd"=w989, "Sample time"=w1027) -> ("dup VISA resource name"=w1006:refnum<visa-resource-name>, "error out"=w1005:errorcluster)  [unwired: 3 in]
        n289 = Number To Decimal String(number=w990) -> (decimal integer string=w1016:string)  [unwired: 1 in]
        n290 = call "4155C Take Sample FPP.vi"("VISA resource name in"=w1006, "error in (no error)"=w1005, "Emergency Stop"=w1007) -> ("Time"=w1011:dbl[], "Vp1"=w1021:dbl[], "VISA Resource Name out"=w987:refnum<visa-resource-name>, "Ig"=w1009:dbl[], "Id"=w1010:dbl[], "Vp2"=w1019:dbl[], "error out"=w1008:errorcluster)  [unwired: 10 in]
        n291 = Insert Into Array(array=dbl[][] [] ("Input Array"), new element=w1011) -> (w1025:dbl[][])  [unwired: 2 in]
        n292 = Number To Decimal String(number=w989) -> (decimal integer string=w1014:string)  [unwired: 1 in]
        n293 = Insert Into Array(array=w1025, new element=w1010) -> (w1024:dbl[][])  [unwired: 2 in]
        n294 = Concatenate Strings("(Vg = " ("Substring"), w1016, "V, Vd = " ("Substring"), w1014, "V)" ("Substring")) -> (w1012:string)
        n295 = Insert Into Array(array=w1024, new element=w1009) -> (w1023:dbl[][])  [unwired: 2 in]
        n296 = Insert Into Array(array=w1023, new element=w1021) -> (w1020:dbl[][])  [unwired: 2 in]
        n297 = Insert Into Array(array=w1020, new element=w1019) -> (w988:dbl[][])  [unwired: 2 in]
        n298 = call <vilib>:"compatOverwrite.vi"("overwrite (F)"=TRUE) -> ("overwrite?"=w985:T7)
        n299 = Open/Create/Replace File(file path (use dialog)=w1004, error in=w1008, operation (0:open)=w985) -> (refnum out=w1001:refnum<file>, error out=w1002:errorcluster)  [unwired: 3 in, 1 out]
        n300 = Array To Spreadsheet String(array=w992, 3:w996) -> (spreadsheet string=w998:string)  [unwired: 1 in]
        n301 = Transpose 2D Array(2D array=w988) -> (transposed array=w1018:dbl[][])
        n302 = Search and Replace String(replace all?=TRUE ("replace all? (F)"), input string=w998, search string="VgVd", replace string=w1012) -> (result string=w994:string)  [unwired: 4 in, 3 out]
        n303 = Spreadsheet String To Array(format string=w996, spreadsheet string=w994, array type (2D Dbl)=w992) -> (array=w993:string[])  [unwired: 1 in]
        n304 = call "4155C Write array to file.vi"("Byte Stream File Refnum"=w1001, "Header"=w993, "Data Array"=w1018, "error in (no error)"=w1002) -> ("dup refnum"=w999:refnum<file>, "error out"=w1000:errorcluster)  [unwired: 1 in]
        n305 = Close File(refnum=w999, error in=w1000) -> (error out=w986:errorcluster)  [unwired: 1 out]
      }
      frame "resample-fpp" {
        w1062 = string[] ["Time /s", "Id VgVd /A", "Ig VgVd /A", "Vp1 VgVd /V", "Vp2 VgVd /V"] ("Header")
        w1066 = "%d" ("format string")
        n306 = Number To Decimal String(number=w1048) -> (decimal integer string=w1106:string)  [unwired: 1 in]
        n307 = Fract/Exp String To Number(string=w1103) -> (number=w1055:dbl[])  [unwired: 3 in, 1 out]
        n308 = Concatenate Strings(w1099, "-resamplefpp-" ("Substring"), w1106, w1049, ".txt" ("Substring")) -> (w1104:string)
        n309 = String To Path(string=w1104) -> (path=w1074:path)
        n310 = Index Array(array=w1055, index=0 ("Index")) -> (element=w1061:dbl)
        n311 = Index Array(array=w1055, index=1 ("Index")) -> (element=w1060:dbl)
        n312 = Number To Decimal String(number=w1061) -> (decimal integer string=w1084:string)  [unwired: 1 in]
        n313 = call "4155C Take Sample FPP.vi"("VISA resource name in"=w1057, "error in (no error)"=w1056, "Emergency Stop"=w1075) -> ("Time"=w1079:dbl[], "Vp1"=w1089:dbl[], "VISA Resource Name out"=w1059:refnum<visa-resource-name>, "Ig"=w1077:dbl[], "Id"=w1078:dbl[], "Vp2"=w1087:dbl[], "error out"=w1076:errorcluster)  [unwired: 10 in]
        n314 = Insert Into Array(array=dbl[][] [] ("Input Array"), new element=w1079) -> (w1093:dbl[][])  [unwired: 2 in]
        n315 = Number To Decimal String(number=w1060) -> (decimal integer string=w1082:string)  [unwired: 1 in]
        n316 = Insert Into Array(array=w1093, new element=w1078) -> (w1092:dbl[][])  [unwired: 2 in]
        n317 = Concatenate Strings("(Vg = " ("Substring"), w1084, "V, Vd = " ("Substring"), w1082, "V)" ("Substring")) -> (w1080:string)
        n318 = Insert Into Array(array=w1092, new element=w1077) -> (w1091:dbl[][])  [unwired: 2 in]
        n319 = Insert Into Array(array=w1091, new element=w1089) -> (w1088:dbl[][])  [unwired: 2 in]
        n320 = Insert Into Array(array=w1088, new element=w1087) -> (w1054:dbl[][])  [unwired: 2 in]
        n321 = call <vilib>:"compatOverwrite.vi"("overwrite (F)"=TRUE) -> ("overwrite?"=w1053:T7)
        n322 = Open/Create/Replace File(file path (use dialog)=w1074, error in=w1076, operation (0:open)=w1053) -> (refnum out=w1071:refnum<file>, error out=w1072:errorcluster)  [unwired: 3 in, 1 out]
        n323 = Array To Spreadsheet String(array=w1062, 3:w1066) -> (spreadsheet string=w1068:string)  [unwired: 1 in]
        n324 = Transpose 2D Array(2D array=w1054) -> (transposed array=w1086:dbl[][])
        n325 = Search and Replace String(replace all?=TRUE ("replace all? (F)"), input string=w1068, search string="VgVd", replace string=w1080) -> (result string=w1064:string)  [unwired: 4 in, 3 out]
        n326 = Spreadsheet String To Array(format string=w1066, spreadsheet string=w1064, array type (2D Dbl)=w1062) -> (array=w1063:string[])  [unwired: 1 in]
        n327 = call "4155C Write array to file.vi"("Byte Stream File Refnum"=w1071, "Header"=w1063, "Data Array"=w1086, "error in (no error)"=w1072) -> ("dup refnum"=w1069:refnum<file>, "error out"=w1070:errorcluster)  [unwired: 1 in]
        n328 = Close File(refnum=w1069, error in=w1070) -> (error out=w1058:errorcluster)  [unwired: 1 out]
      }
      frame "serial" {
        n329 = Index Array(array=w1110, index=0 ("Index")) -> (element=w1109:string)
        n330 = call "Serial write and read v0.4.vi"("Termination char\n(0xA = '\\n' = LF)\n(0xD = '\\r' = CR)"="Termination char\n(0xA = '\\n' = LF)\n(0xD = '\\r' = CR)", "Enable Termination\nChar (T)"="Enable Termination\nChar (T)", "parity"="parity", "stop bits"="stop bits", "string to write"=w1109, "flow control"="flow control", "byte count"="byte count", "Serial Settings:Serial End Mode for Reads"="Serial Settings:Serial End Mode for Reads", "Timeout (ms)"="Timeout (ms)", "error in (no error)"=w1115, "VISA resource name"="VISA resource name", "baud rate"="baud rate", "data bits"="data bits") -> ("read string"=→"Serial output":string, "error out"=w1114:errorcluster)  [unwired: 1 in]
      }
    }
  }
  "error out" <- w9
